vi "TEST.vi"() -> ()   [LabVIEW 2021]
uses:
  TEST ENNUM.ctl
  <vilib>/Instr/_visa.llb/VISA Configure Serial Port (Instr).vi
  <vilib>/Utility/file.llb/Write Delimited Spreadsheet (string).vi
  <vilib>/Utility/config.llb/NI_LVConfig.lvlib
  <vilib>/Utility/miscctls.llb/LVPointTypeDef.ctl
  Settings page.vi
  Exit Variable.vi
  Control 4.ctl
  <vilib>/Utility/config.llb/Write Key (Double).vi
panel:
  out "Printer":bool
  out "Part ID":string
  out "Printer Command":string
  out "TETS TYPE":string
  out "TETS MODE":string
  in  "Exit Button":bool
  in  "SETTINGS BUTTON 2":bool
  out "Communication Status":bool
  out "CH 1 FAIL":bool
  out "CH 10 FAIL":bool
  out "CH 10  PASS":bool
  out "CH 5 FAIL":bool
  out "CH 5 PASS":bool
  out "CH 4 FAIL":bool
  out "CH 4 PASS":bool
  out "CH 9 FAIL":bool
  out "CH 9 PASS":bool
  out "CH 8 FAIL":bool
  out "CH 8 PASS":bool
  out "CH 3 FAIL":bool
  out "CH 3 PASS":bool
  out "CH 2 FAIL":bool
  out "CH 2 PASS":bool
  out "CH 7 FAIL":bool
  out "CH 7 PASS":bool
  out "CH 6 FAIL":bool
  out "CH 6 PASS":bool
  out "CH 1 PASS":bool
  out "CH 10 RES VAL":string
  out "CH 10 STATUS":string
  out "CH 9 RES VAL":string
  out "CH 9 STATUS":string
  out "CH 8 RES VAL":string
  out "CH 8 STATUS":string
  out "CH 7 RES VAL":string
  out "CH 7 STATUS":string
  out "CH 6 RES VAL":string
  out "CH 6 STATUS":string
  out "CH 5 RES VAL":string
  out "CH 5 STATUS":string
  out "CH 4 RES VAL":string
  out "CH 4 STATUS":string
  out "CH 3 RES VAL":string
  out "CH 3 STATUS":string
  out "CH 2 RES VAL":string
  out "CH 2 STATUS":string
  out "Cancel Button":bool
  out "CH 1 RES VAL":string
  out "CH1 STATUS":string
  # "EOL TEST BENCH FOR THERMISTOR"
  # "Communication Status"
  # "Printer Communication Status"
  # "CHANNEL 5"
  # "CHANNEL 3"
  # "CHANNEL 4"
  # "CHANNEL 1"
  # "CHANNEL 2"
  # "STATUS"
  # "STATUS"
  # "STATUS"
  # "STATUS"
  # "STATUS"
  # "k Ohm"
  # "k Ohm"
  # "RESISTANCE VALUE"
  # "RESISTANCE VALUE"
  # "RESISTANCE VALUE"
  # "k Ohm"
  # "RESISTANCE VALUE"
  # "k Ohm"
  # "RESISTANCE VALUE"
  # "k Ohm"
  # "PASS"
  # "FAIL"
  # "PASS"
  # "FAIL"
  # "PASS"
  # "FAIL"
  # "PASS"
  # "FAIL"
  # "PASS"
  # "FAIL"
  # "QR DATA"
  # "CHANNEL 7"
  # "CHANNEL 6"
  # "CHANNEL 10"
  # "CHANNEL 8"
  # "CHANNEL 9"
  # "STATUS"
  # "STATUS"
  # "STATUS"
  # "STATUS"
  # "STATUS"
  # "RESISTANCE VALUE"
  # "RESISTANCE VALUE"
  # "k Ohm"
  # "RESISTANCE VALUE"
  # "k Ohm"
  # "RESISTANCE VALUE"
  # "k Ohm"
  # "k Ohm"
  # "RESISTANCE VALUE"
  # "k Ohm"
  # "PASS"
  # "FAIL"
  # "PASS"
  # "FAIL"
  # "PASS"
  # "FAIL"
  # "PASS"
  # "FAIL"
  # "PASS"
  # "FAIL"
  # "MODE :"
  # "TEST TYPE :"
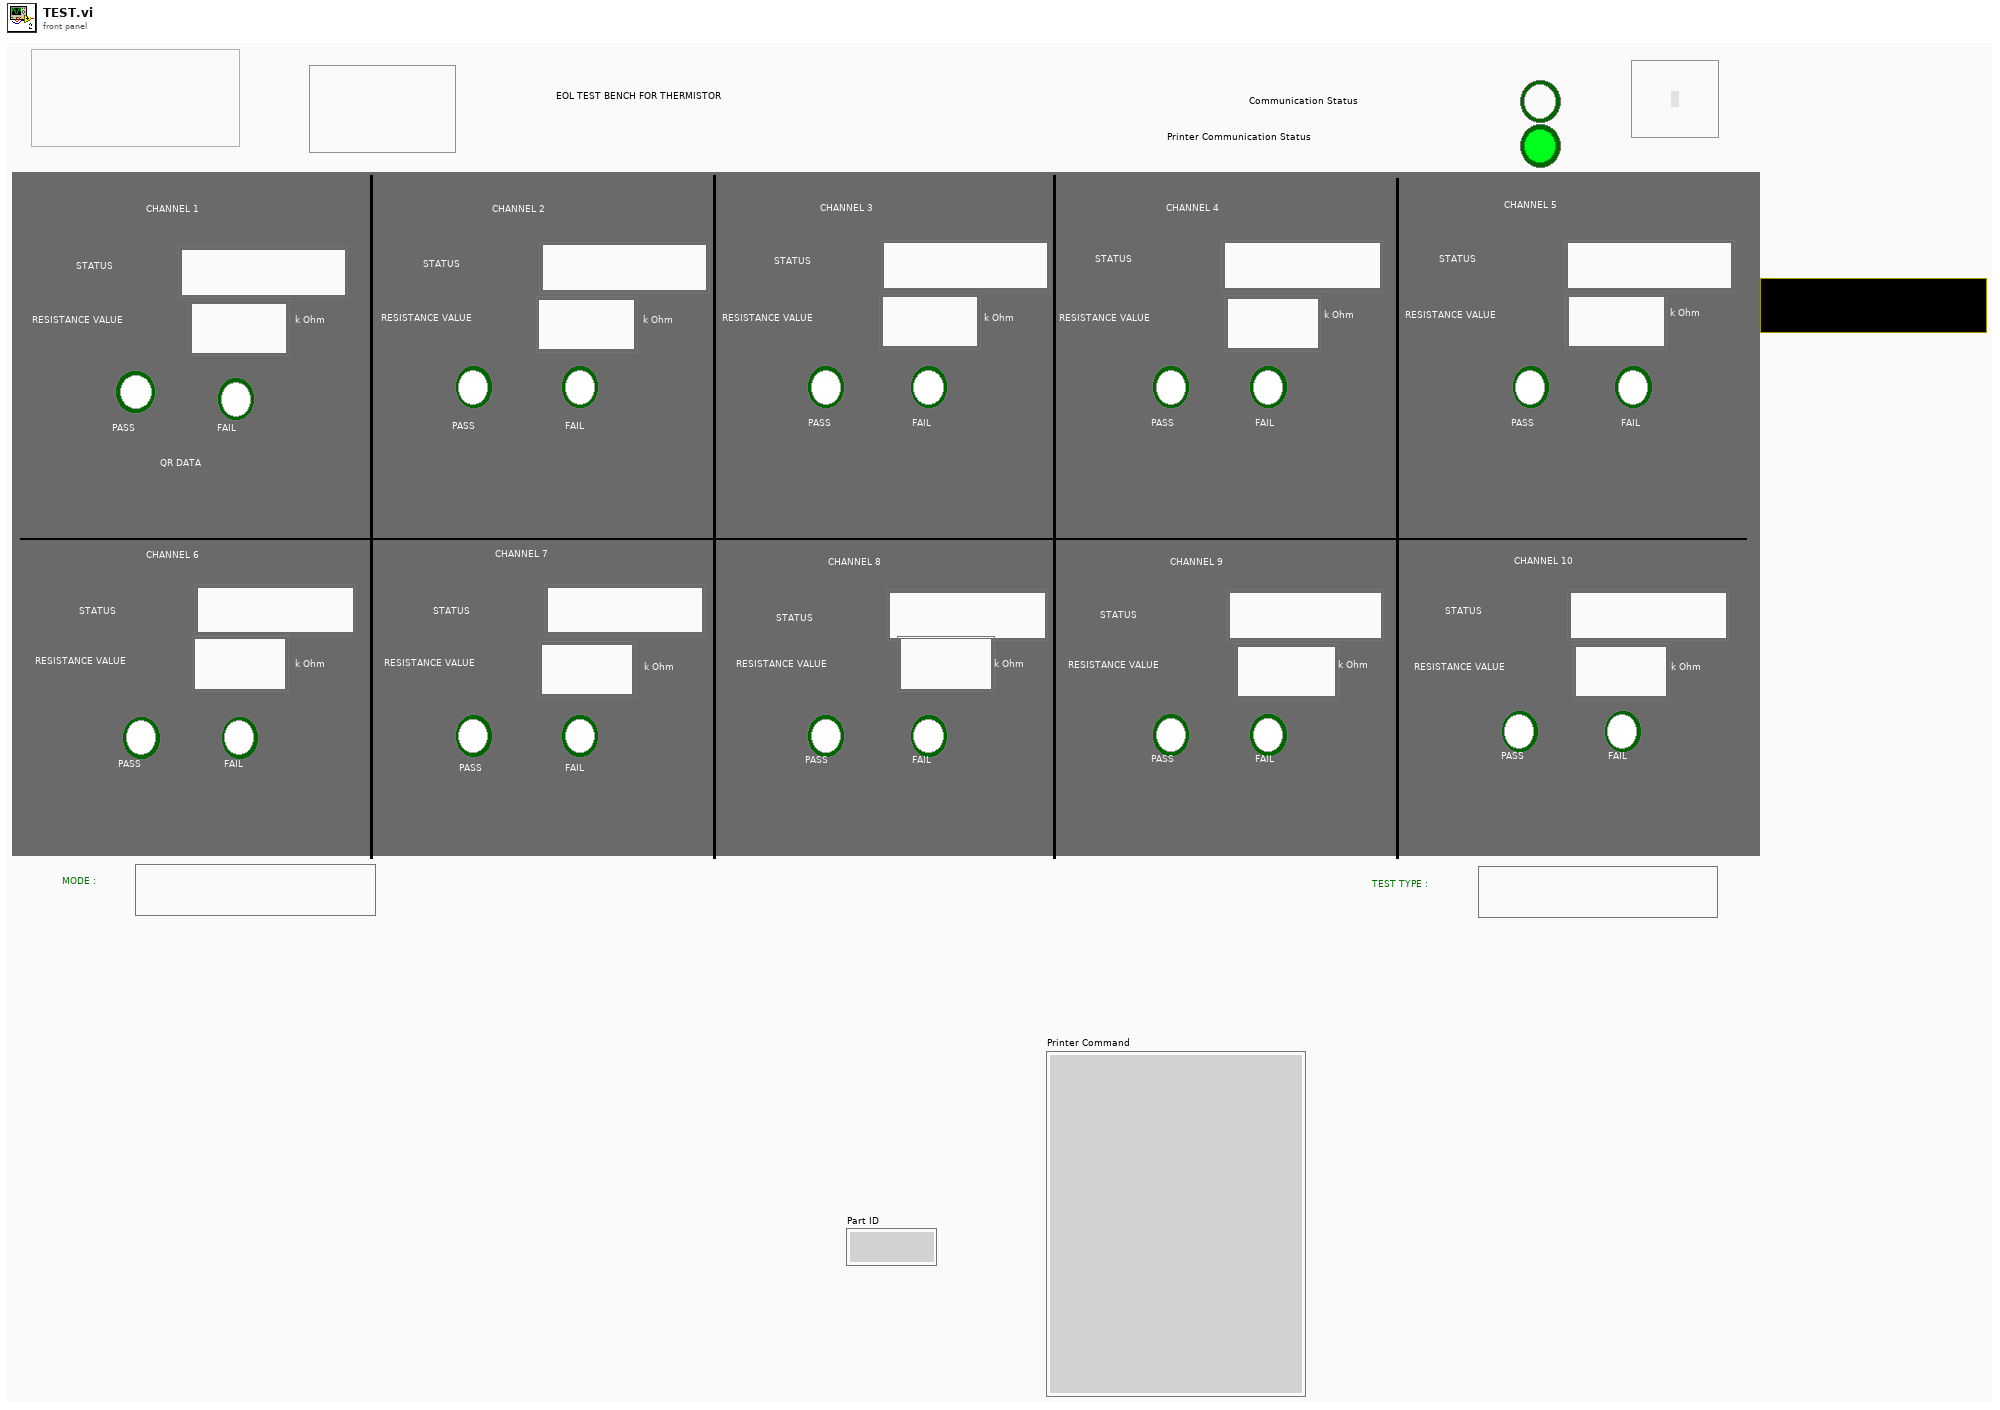
[diagram p1: front panel]
types:
  T1 = typedef "LVPointTypeDef.ctl" = cluster{"Horizontal":i16, "Vertical":i16}
  T2 = typedef "Control 4.ctl" = cluster{"VISA resource name":refnum<visa-resource-name>, "MODE":string, "PP 1":i32, "PP 2":i32, "PP 3":i32, "PP 4":i32, "PP 5":i32, "PP 6":i32, "PP 7":i32, "PP 8":i32, "PP 9":i32, "PP 10":i32, "CH  PASS  1":bool, "CH  PASS 2":bool, "CH  PASS 3":bool, "CH  PASS 4":bool, "CH  PASS 5":bool, "CH  PASS 6":bool, "CH  PASS 7":bool, "CH  PASS 8":bool, "CH  PASS 9":bool, "CH  PASS 10":bool, "CH  FAIL 1":bool, "CH  FAIL 2":bool, "CH  FAIL 3":bool, "CH  FAIL 4":bool, "CH  FAIL 5":bool, "CH  FAIL 6":bool, "CH  FAIL 7":bool, "CH  FAIL 8":bool, "CH  FAIL 9":bool, "CH  FAIL 10":bool, "RES VALUE 1":dbl, "RES VALUE 2":dbl, "RES VALUE 3":dbl, "RES VALUE 4":dbl, "RES VALUE 5":dbl, "RES VALUE 6":dbl, "RES VALUE 7":dbl, "RES VALUE 8":dbl, "RES VALUE 9":dbl, "RES VALUE 10":dbl, "SET VALUE 1":dbl, "SET VALUE 2":dbl, "SET VALUE 3":dbl, "SET VALUE 4":dbl, "SET VALUE 5":dbl, "SET VALUE 6":dbl, "SET VALUE 7":dbl, "SET VALUE 8":dbl, "SET VALUE 9":dbl, "SET VALUE 10":dbl, "TOL 1":dbl, "TOL 2":dbl, "TOL 3":dbl, "TOL 4":dbl, "TOL 5":dbl, "TOL 6":dbl, "TOL 7":dbl, "TOL 8":dbl, "TOL 9":dbl, "TOL 10":dbl, "START BIT":i32, "CH1 MIN TOL":dbl, "CH2 MIN TOL ":dbl, "CH3 MIN TOL ":dbl, "CH4 MIN TOL ":dbl, "CH5 MIN TOL ":dbl, "CH6 MIN TOL ":dbl, "CH7 MIN TOL  ":dbl, "CH8 MIN TOL  ":dbl, "CH9 MIN TOL   ":dbl, "CH10 MIN TOL   ":dbl, "CH1 MAX TOL ":dbl, "CH2 MAX TOL  ":dbl, "CH3 MAX TOL  ":dbl, "CH4 MAX TOL ":dbl, "CH5 MAX TOL  ":dbl, "CH6 MAX TOL  ":dbl, "CH7 MAX TOL   ":dbl, "CH8 MAX TOL  ":dbl, "CH9 MAX TOL    ":dbl, "CH10 MAX TOL   ":dbl}
  T3 = typedef "TEST ENNUM.ctl" = enum16{"TIMEOUT", "INITIALIZE", "CH SELECTION", "VALIDATING", "RESULT", "LED_SEQ", "READY TO PRINT", "REPORT ", "PART PRESENCE CHECKING"}
  T4 = typedef "NI_LVConfig.lvlib/Config Data RefNum.ctl" = refnum<k1>
  T5 = typedef "SERIAL N0.ctl" = string
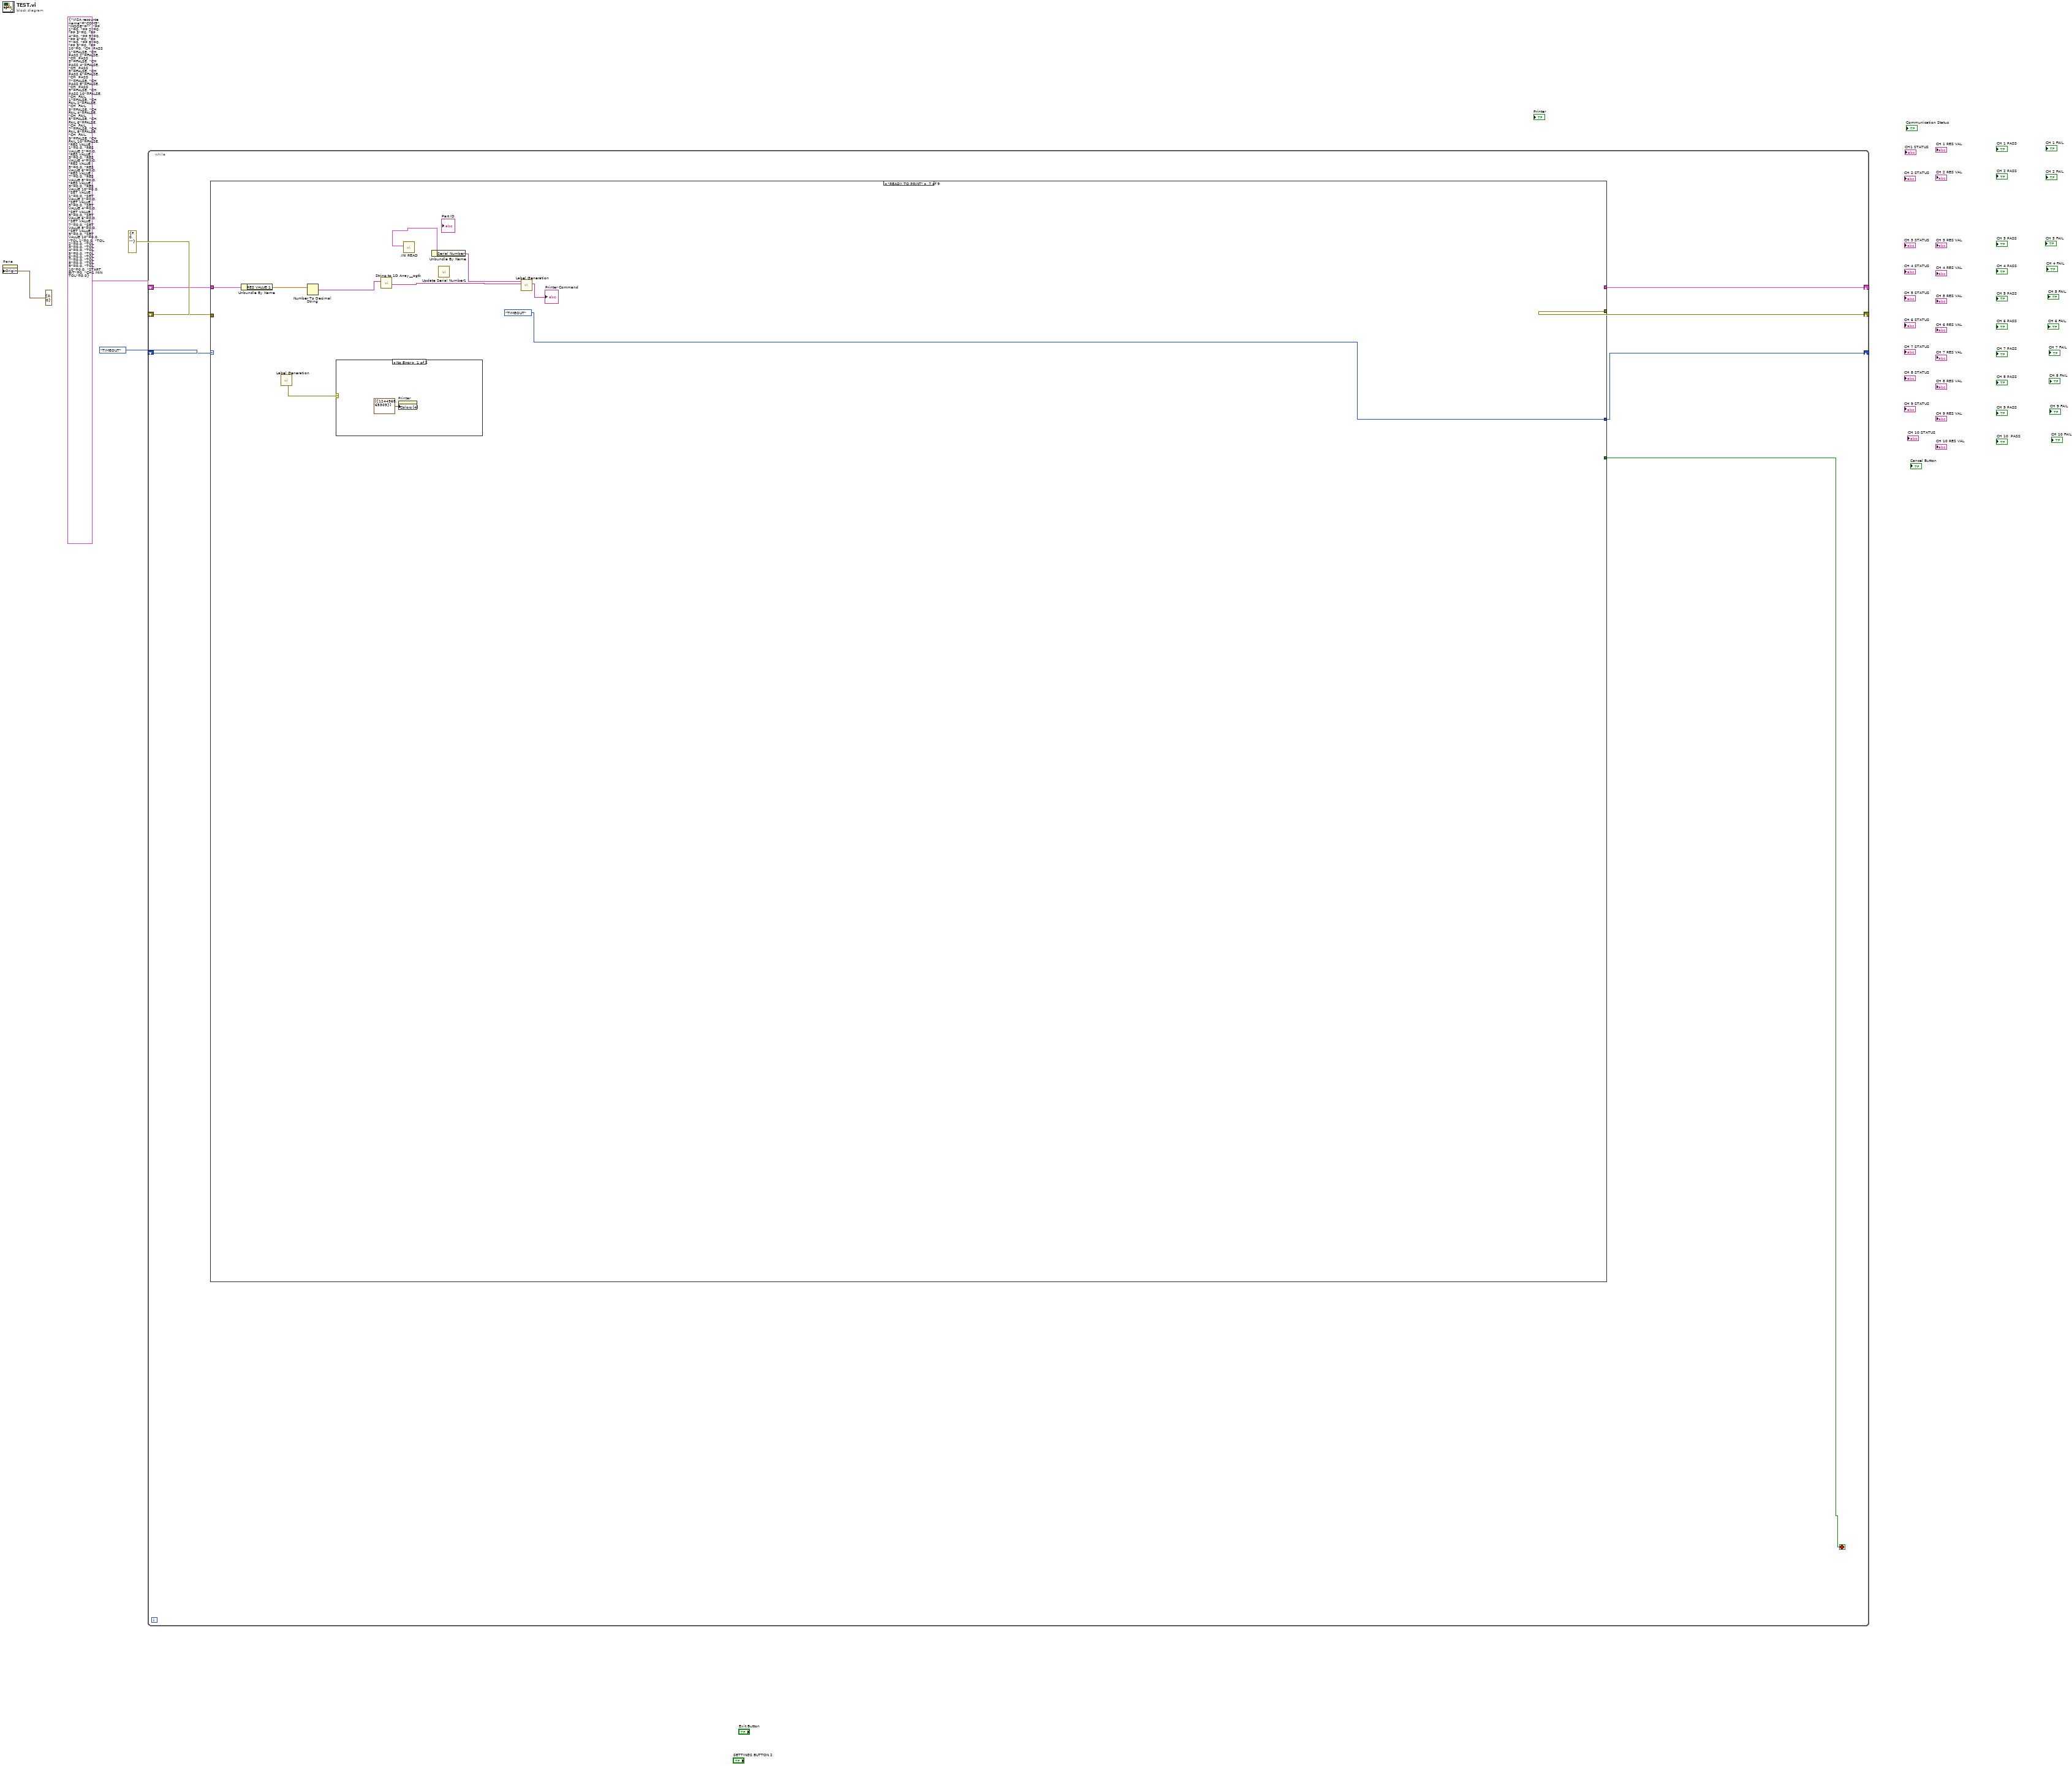
[diagram p0: block diagram]
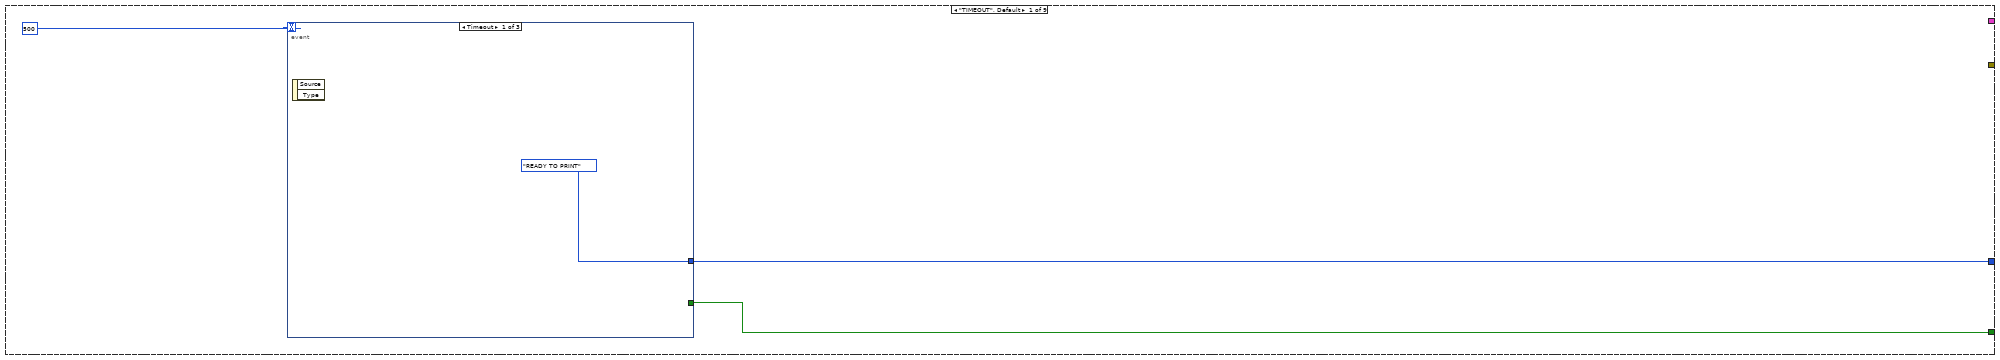
[diagram p2: hidden frame]
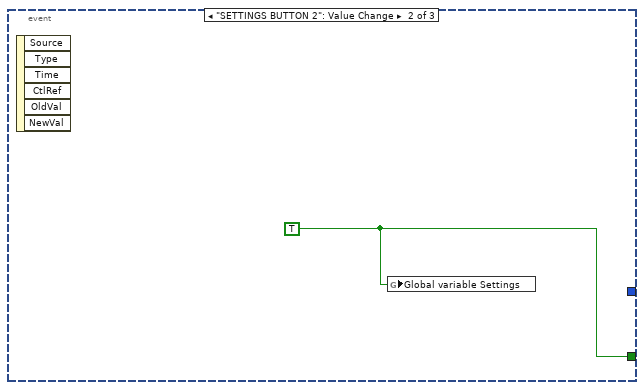
[diagram p3: hidden frame]
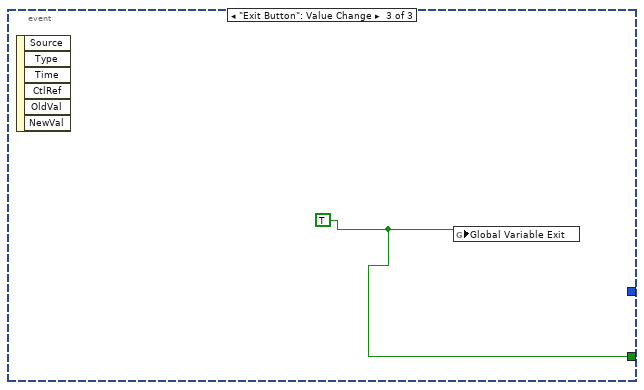
[diagram p4: hidden frame]
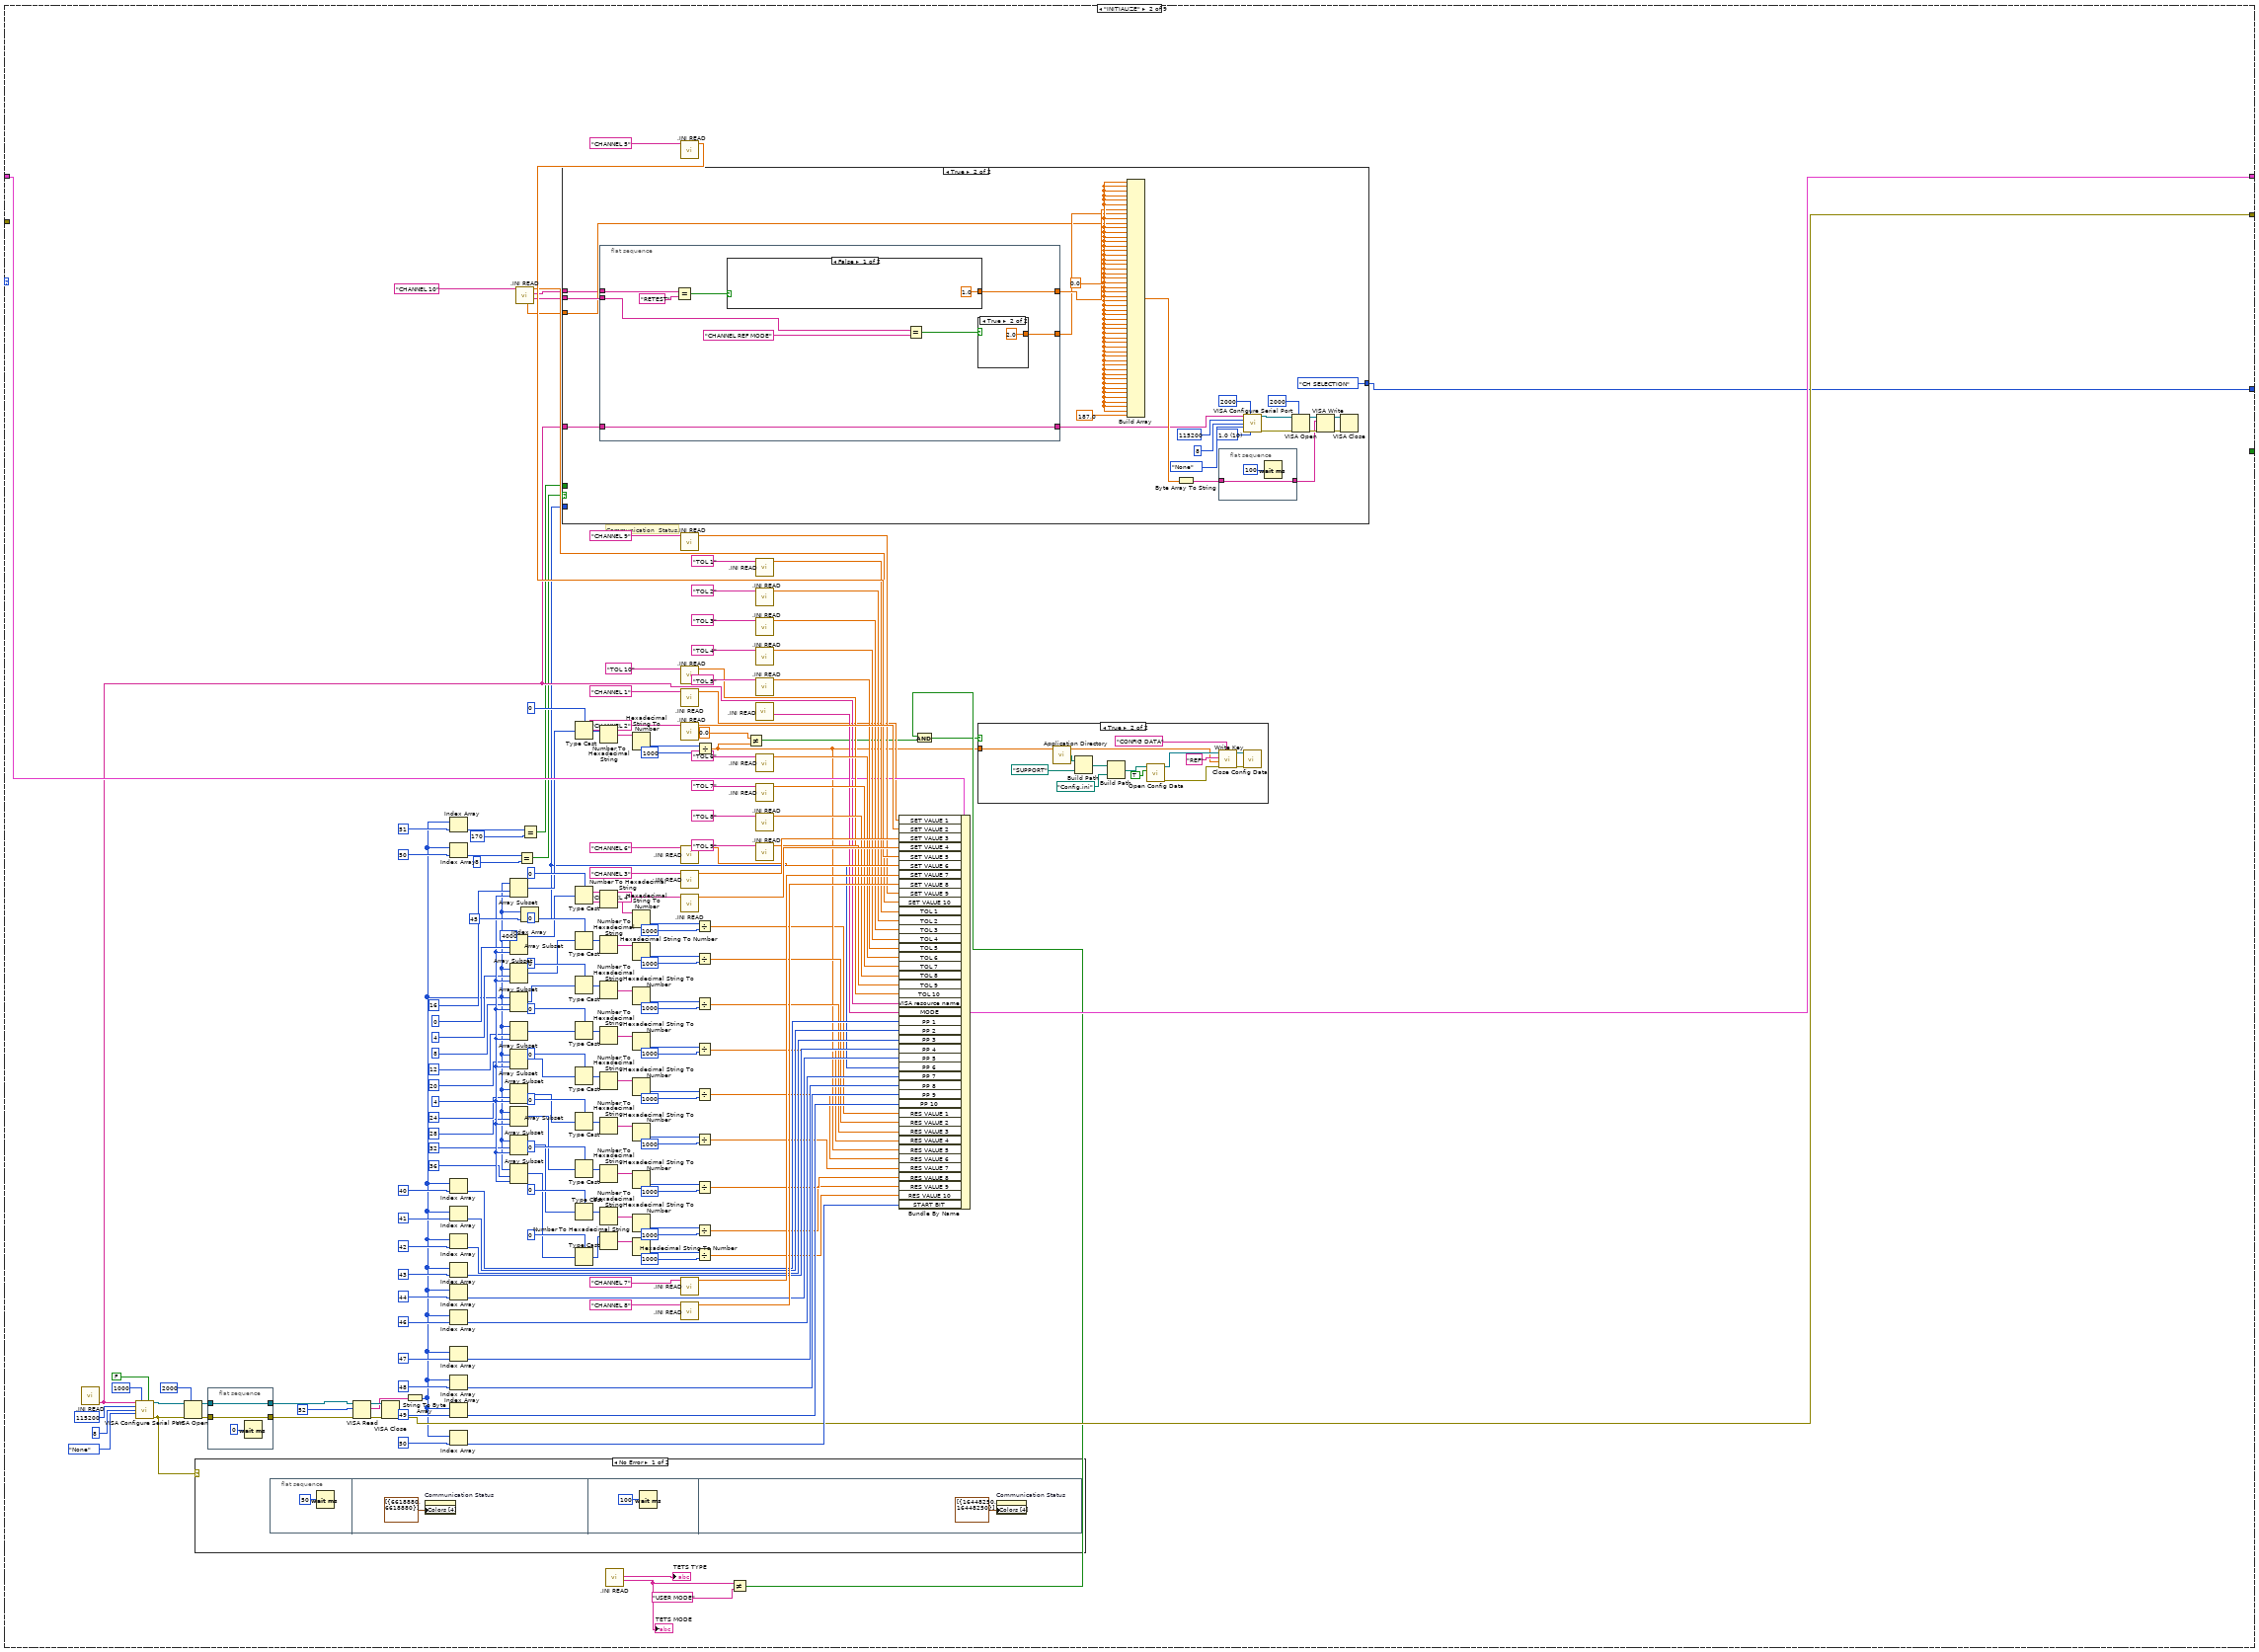
[diagram p5: hidden frame]
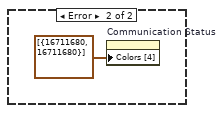
[diagram p7: hidden frame]
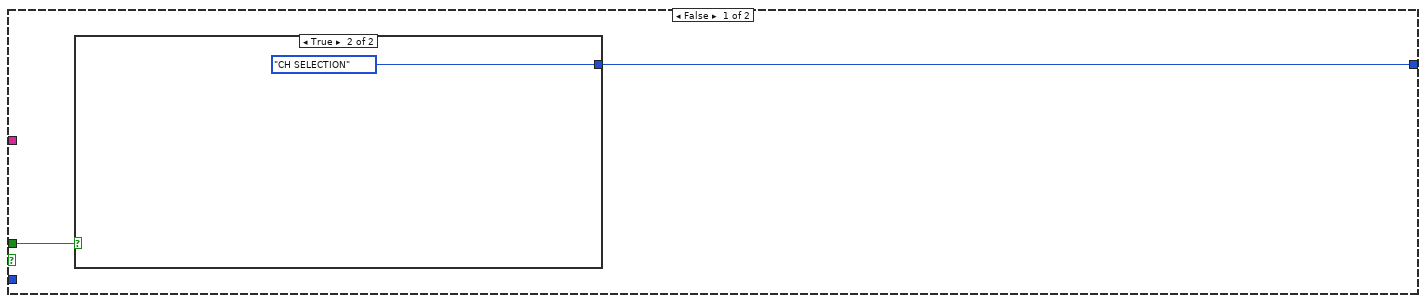
[diagram p8: hidden frame]
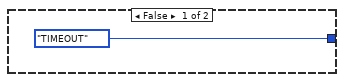
[diagram p9: hidden frame]
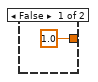
[diagram p10: hidden frame]
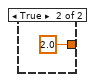
[diagram p11: hidden frame]
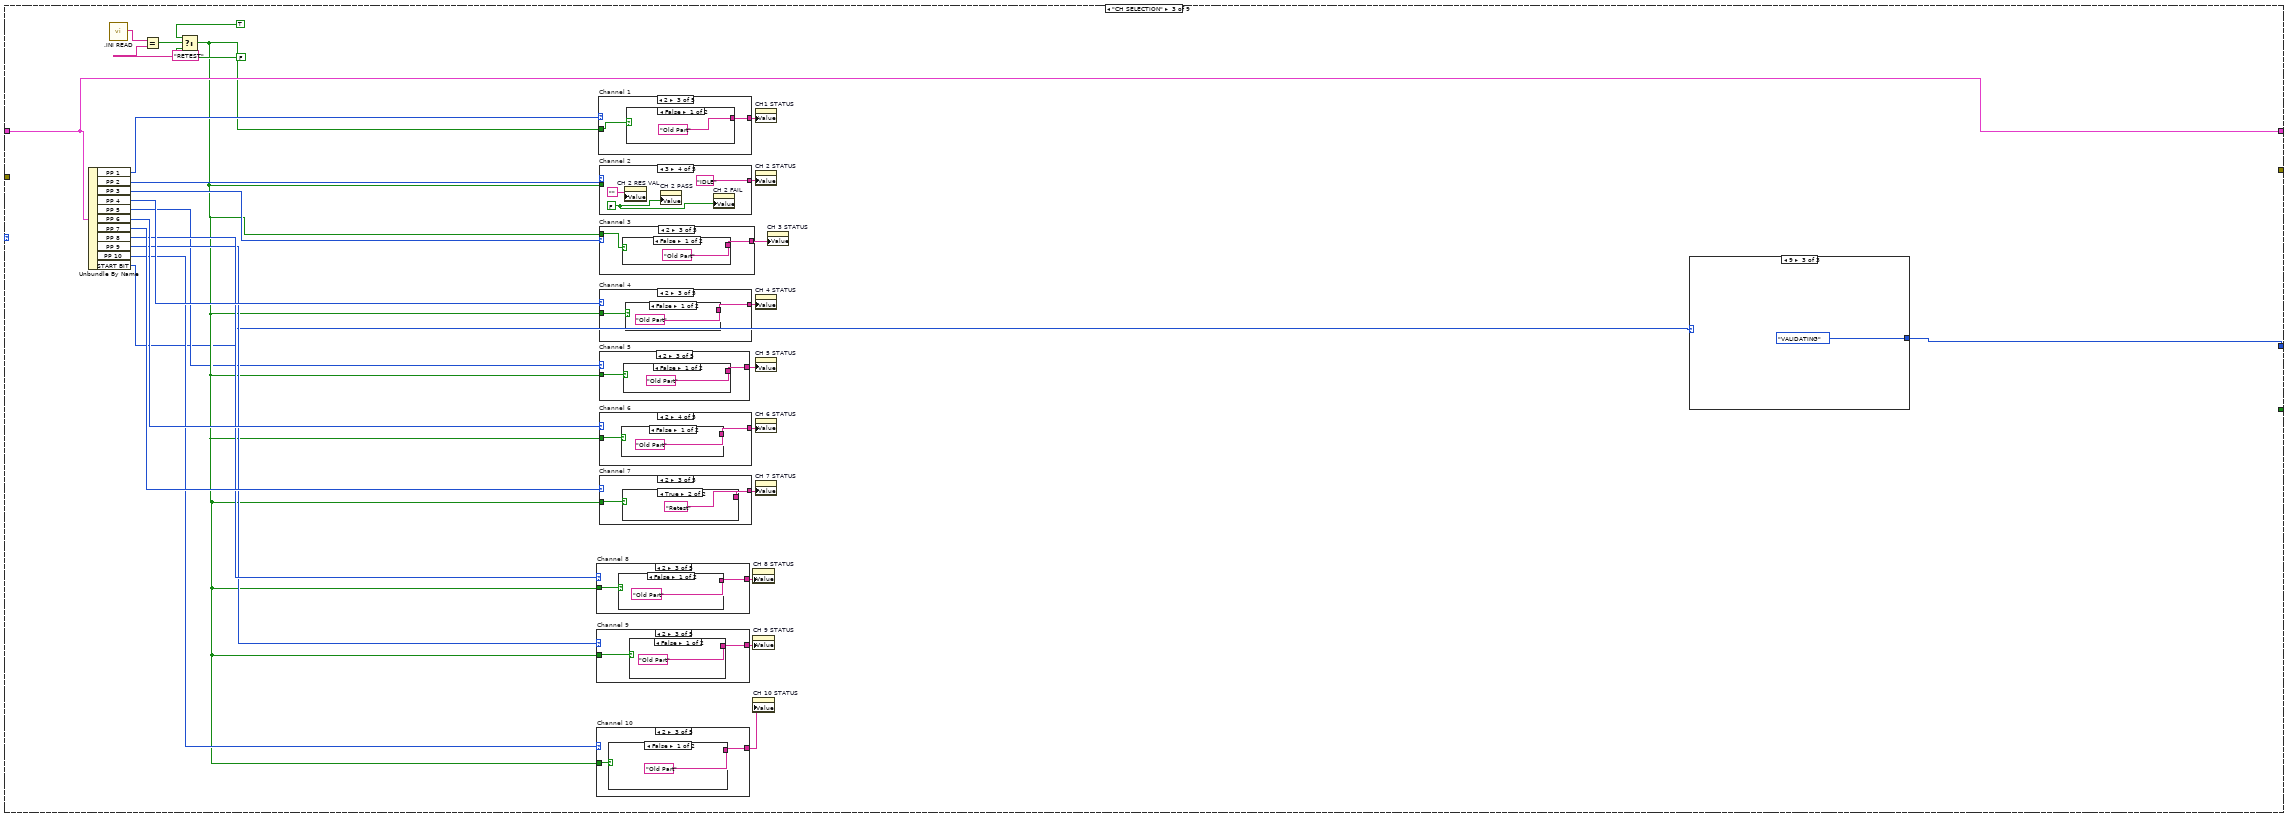
[diagram p12: hidden frame]
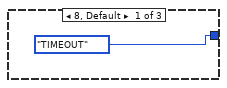
[diagram p13: hidden frame]
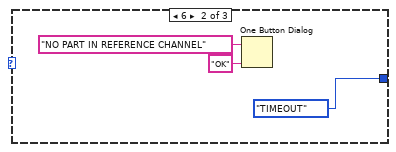
[diagram p14: hidden frame]
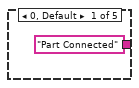
[diagram p15: hidden frame]
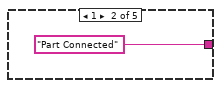
[diagram p16: hidden frame]
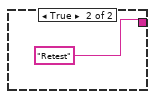
[diagram p17: hidden frame]
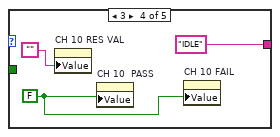
[diagram p18: hidden frame]
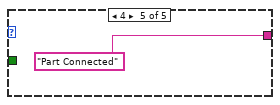
[diagram p19: hidden frame]
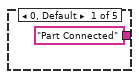
[diagram p20: hidden frame]
diagram:
  n1 = property on="Pane" class="Pane"("Origin"=T1 {"Horizontal"=0, "Vertical"=0}) -> ()  [unwired: 2 in, 2 out]
  n2 = while {
    shift-right: [w10] -> _
    shift-left: TEST_ENNUM."TIMEOUT" -> [w11]
    shift-right: [w9] -> _
    shift-left: T2 {"VISA resource name"="COM5", "MODE"="", "PP 1"=0, "PP 2"=0, "PP 3"=0, "PP 4"=0, "PP 5"=0, "PP 6"=0, "PP 7"=0, "PP 8"=0, "PP 9"=0, "PP 10"=0, "CH  PASS  1"=FALSE, "CH  PASS 2"=FALSE, "CH  PASS 3"=FALSE, "CH  PASS 4"=FALSE, "CH  PASS 5"=FALSE, "CH  PASS 6"=FALSE, "CH  PASS 7"=FALSE, "CH  PASS 8"=FALSE, "CH  PASS 9"=FALSE, "CH  PASS 10"=FALSE, "CH  FAIL 1"=FALSE, "CH  FAIL 2"=FALSE, "CH  FAIL 3"=FALSE, "CH  FAIL 4"=FALSE, "CH  FAIL 5"=FALSE, "CH  FAIL 6"=FALSE, "CH  FAIL 7"=FALSE, "CH  FAIL 8"=FALSE, "CH  FAIL 9"=FALSE, "CH  FAIL 10"=FALSE, "RES VALUE 1"=0.0, "RES VALUE 2"=0.0, "RES VALUE 3"=0.0, "RES VALUE 4"=0.0, "RES VALUE 5"=0.0, "RES VALUE 6"=0.0, "RES VALUE 7"=0.0, "RES VALUE 8"=0.0, "RES VALUE 9"=0.0, "RES VALUE 10"=0.0, "SET VALUE 1"=0.0, "SET VALUE 2"=0.0, "SET VALUE 3"=0.0, "SET VALUE 4"=0.0, "SET VALUE 5"=0.0, "SET VALUE 6"=0.0, "SET VALUE 7"=0.0, "SET VALUE 8"=0.0, "SET VALUE 9"=0.0, "SET VALUE 10"=0.0, "TOL 1"=0.0, "TOL 2"=0.0, "TOL 3"=0.0, "TOL 4"=0.0, "TOL 5"=0.0, "TOL 6"=0.0, "TOL 7"=0.0, "TOL 8"=0.0, "TOL 9"=0.0, "TOL 10"=0.0, "START BIT"=0, "CH1 MIN TOL"=0.0, "CH2 MIN TOL "=0.0, "CH3 MIN TOL "=0.0, "CH4 MIN TOL "=0.0, "CH5 MIN TOL "=0.0, "CH6 MIN TOL "=0.0, "CH7 MIN TOL  "=0.0, "CH8 MIN TOL  "=0.0, "CH9 MIN TOL   "=0.0, "CH10 MIN TOL   "=0.0, "CH1 MAX TOL "=0.0, "CH2 MAX TOL  "=0.0, "CH3 MAX TOL  "=0.0, "CH4 MAX TOL "=0.0, "CH5 MAX TOL  "=0.0, "CH6 MAX TOL  "=0.0, "CH7 MAX TOL   "=0.0, "CH8 MAX TOL  "=0.0, "CH9 MAX TOL    "=0.0, "CH10 MAX TOL   "=0.0} ("Cluster") -> [w7]
    shift-right: [w8] -> _
    shift-left: errorcluster {"status"=FALSE, "code"=0, "source"=""} ("error out") -> [w6]
    stop <- w5 stop-if-true
    n3 = case shown="\"READY TO PRINT\"" w11 {
      tunnel: [w13 w55 w267 TEST_ENNUM."RESULT" TEST_ENNUM."LED_SEQ" TEST_ENNUM."READY TO PRINT" TEST_ENNUM."TIMEOUT" TEST_ENNUM."TIMEOUT" _] -> w10
      tunnel: w7 -> [_ w141 w276 w423 w643 w862 w1024 w1035 _]
      tunnel: [_ w142 w276 w536 w643 w862 _ _ _] -> w9
      tunnel: [_ w59 _ _ _ w860 _ _ _] -> w8
      tunnel: w6 -> [_ _ _ _ _ _ _ _ _]
      tunnel: [w12 _ _ _ _ _ _ _ _] -> w5
      frame "TIMEOUT", Default {
        n4 = event shown="[0] Timeout" {
          selector: _ -> [_ _ _]
          dyn-events: _ -> [_ _ _]
          timeout: 500 -> [_ _ _]
          tunnel: [_ w16 w17] -> w12
          tunnel: [TEST_ENNUM."READY TO PRINT" _ _] -> w13
          event Timeout {
            n5 = event-data() -> ()  [unwired: 1 in, 2 out]
          }
          event "SETTINGS BUTTON 2": Value Change {
            w16 = TRUE
            n6 = event-data() -> ()  [unwired: 1 in, 6 out]
            n7 = global write "Settings page.vi" "Global variable Settings"(w16) -> ()
          }
          event "Exit Button": Value Change {
            w17 = TRUE
            n8 = event-data() -> ()  [unwired: 1 in, 6 out]
            n9 = global write "Exit Variable.vi" "Global Variable Exit"(w17) -> ()
          }
        }
      }
      frame "INITIALIZE" {
        w139 = 4 ("length")
        # "Communication  Status"
        n10 = call ".INI READ.vi"() -> ("COM"=w56:string)  [unwired: 4 in, 7 out]
        n11 = call-poly "VISA Configure Serial Port"("VISA resource name"=w56, "timeout (10sec)"=u32 1000, "Enable Termination\nChar (T)"=FALSE ("Enable Termination\nChar (T)"), "baud rate (9600)"=u32 115200, "data bits (8)"=u16 8, "parity (0:none)"=enum16{"None", "Odd", "Even", "Mark", "Space"}."None") -> ("VISA resource name out"=w46:refnum<visa-resource-name>, "error out"=w61:errorcluster)  [unwired: 8 in]
        n12 = VISA Open(timeout (0)=u32 2000 ("VISA Open timeout (0)"), error in (no error)=w61, VISA resource name=w46) -> (VISA resource name=w38:refnum<visa-resource-name>, error out=w40:errorcluster)  [unwired: 2 in]
        n13 = case shown="No Error" w61 {
          frame No Error {
            n14 = flat-sequence {
              frame #0 {
                n15 = Wait (ms)(milliseconds to wait=u32 50) -> ()  [unwired: 1 out]
              }
              frame #1 {
                n16 = property on="Communication Status" class="Bool (strict)"("Colors [4]"=cluster{u32, u32}[] [{6618880, 6618880}]) -> ()  [unwired: 2 in, 2 out]
              }
              frame #2 {
                n17 = Wait (ms)(milliseconds to wait=u32 100) -> ()  [unwired: 1 out]
              }
              frame #3 {
                n18 = property on="Communication Status" class="Bool (strict)"("Colors [4]"=cluster{u32, u32}[] [{16448250, 16448250}]) -> ()  [unwired: 2 in, 2 out]
              }
            }
          }
          frame Error {
            n19 = property on="Communication Status" class="Bool (strict)"("Colors [4]"=cluster{u32, u32}[] [{16711680, 16711680}]) -> ()  [unwired: 2 in, 2 out]
          }
        }
        n20 = flat-sequence {
          tunnel: [w217] -> w41
          tunnel: w40 -> [w217]
          tunnel: [w216] -> w39
          tunnel: w38 -> [w216]
          frame #0 {
            n21 = Wait (ms)(milliseconds to wait=u32 0) -> ()  [unwired: 1 out]
          }
        }
        n22 = VISA Read(VISA resource name=w39, byte count=u32 52, error in (no error)=w41) -> (VISA resource name out=w42:refnum<visa-resource-name>, read buffer=w36:string, error out=w37:errorcluster)  [unwired: 1 out]
        n23 = VISA Close(VISA resource name=w42, error in (no error)=w37) -> (error out=w59:errorcluster)
        n24 = String To Byte Array(string=w36) -> (unsigned byte array=w28:u8[])
        n25 = Index Array(array=w28, index=51) -> (element=w57:u8)
        n26 = Index Array(array=w28, index=50) -> (element=w52:u8)
        n27 = Index Array(array=w28, index=40) -> (element=w151:u8)
        n28 = Index Array(array=w28, index=41) -> (element=w150:u8)
        n29 = Index Array(array=w28, index=42) -> (element=w149:u8)
        n30 = Index Array(array=w28, index=43) -> (element=w148:u8)
        n31 = Index Array(array=w28, index=44) -> (element=w147:u8)
        n32 = Index Array(array=w28, index=46) -> (element=w146:u8)
        n33 = Index Array(array=w28, index=47) -> (element=w145:u8)
        n34 = Index Array(array=w28, index=48) -> (element=w144:u8)
        n35 = Index Array(array=w28, index=49) -> (element=w143:u8)
        n36 = Index Array(array=w28, index=50) -> (element=w60:u8)
        n37 = Array Subset(array=w28, index=16, length=w139) -> (w109:u8[])
        n38 = Array Subset(array=w28, index=0, length=w139) -> ()  [unwired: 1 out]
        n39 = Array Subset(array=w28, index=4, length=w139) -> (w117:u8[])
        n40 = Array Subset(array=w28, index=8, length=w139) -> (w18:u8[])
        n41 = Array Subset(array=w28, index=12, length=w139) -> (w112:u8[])
        n42 = Array Subset(array=w28, index=20, length=w139) -> (w106:u8[])
        n43 = Array Subset(array=w28, index=24, length=w139) -> (w103:u8[])
        n44 = Array Subset(array=w28, index=28, length=w139) -> (w100:u8[])
        n45 = Array Subset(array=w28, index=32, length=w139) -> (w97:u8[])
        n46 = Array Subset(array=w28, index=36, length=w139) -> (w94:u8[])
        n47 = call ".INI READ.vi"("KEY"="CHANNEL 10") -> ("MODE"=w24:string, "TEST MODE"=w23:string, "OUT"=w183:dbl, "TIME"=w25:dbl)  [unwired: 3 in, 4 out]
        n48 = Equal?(x=w52, y=u8 8) -> (x = y?=w50:bool)
        n49 = Index Array(array=w28, index=45) -> (element=w26:u8)
        n50 = Equal?(x=w57, y=u8 170) -> (x = y?=w53:bool)
        n51 = case shown="True" w50 {
          tunnel: w56 -> [_ w231]
          tunnel: [w223 TEST_ENNUM."CH SELECTION"] -> w55
          tunnel: w53 -> [w224 _]
          tunnel: w26 -> [_ _]
          tunnel: w24 -> [_ w229]
          tunnel: w25 -> [_ w228]
          tunnel: w23 -> [_ w227]
          frame False {
            n52 = case shown="True" w224 {
              tunnel: [TEST_ENNUM."TIMEOUT" TEST_ENNUM."CH SELECTION"] -> w223
              frame False {
              }
              frame True {
              }
            }
          }
          frame True {
            w244 = u16 10 items=["1.0"=10, "1.5"=15, "2.0"=20] ("stop bits (10: 1 bit)")
            w235 = 0.0 ("element")
            n53 = flat-sequence {
              tunnel: [w258] -> w233
              tunnel: [w255] -> w232
              tunnel: w231 -> [w254]
              tunnel: [w254] -> w230
              tunnel: w229 -> [w253]
              tunnel: w227 -> [w252]
              frame #0 {
                n54 = Equal?(x=w252, y="RETEST") -> (x = y?=w259:bool)
                n55 = case shown="False" w259 {
                  tunnel: [1.0 ("element") 2.0 ("element")] -> w258
                  frame False {
                  }
                  frame True {
                  }
                }
                n56 = Equal?(x=w253, y="CHANNEL REF MODE") -> (x = y?=w256:bool)
                n57 = case shown="True" w256 {
                  tunnel: [1.0 ("element") 2.0 ("element")] -> w255
                  frame False {
                  }
                  frame True {
                  }
                }
              }
            }
            n58 = Build Array(w235, w235, w235, w235, w235, w235, w233, w232, w235, w228, w235, w235, w235, w235, w235, w235, w235, w235, w235, w235, w235, w235, w235, w235, w235, w235, w235, w235, w235, w235, w235, w235, w235, w235, w235, w235, w235, w235, w235, w235, w235, w235, w235, w235, w235, w235, w235, w235, w235, w235, w235, 187.0 ("element")) -> (w251:dbl[])
            n59 = Byte Array To String(unsigned byte array=w251) -> (string=w237:string)
            n60 = flat-sequence {
              tunnel: w237 -> [w266]
              tunnel: [w266] -> w236
              frame #0 {
                n61 = Wait (ms)(milliseconds to wait=u32 100) -> ()  [unwired: 1 out]
              }
            }
            n62 = call-poly "VISA Configure Serial Port"("VISA resource name"=w230, "timeout (10sec)"=u32 2000, "baud rate (9600)"=u32 115200, "data bits (8)"=u16 8, "parity (0:none)"=enum16{"None", "Odd", "Even", "Mark", "Space"}."None", "stop bits (10: 1 bit)"=w244) -> ("VISA resource name out"=w250:refnum<visa-resource-name>, "error out"=w249:errorcluster)  [unwired: 8 in]
            n63 = VISA Open(timeout (0)=u32 2000 ("VISA Open timeout (0)"), error in (no error)=w249, VISA resource name=w250) -> (VISA resource name=w243:refnum<visa-resource-name>, error out=w242:errorcluster)  [unwired: 2 in]
            n64 = VISA Write(VISA resource name=w243, write buffer=w236, error in (no error)=w242) -> (VISA resource name out=w240:refnum<visa-resource-name>, error out=w239:errorcluster)  [unwired: 1 out]
            n65 = VISA Close(VISA resource name=w240, error in (no error)=w239) -> ()  [unwired: 1 out]
          }
        }
        n66 = Type Cast(type=0 ("index"), x=w109) -> (*(type *) &x=w108:i32)
        n67 = Type Cast(type=0 ("index"), x=4000) -> (*(type *) &x=w119:i32)
        n68 = Type Cast(type=0 ("index"), x=w117) -> (*(type *) &x=w116:i32)
        n69 = Type Cast(type=0 ("index"), x=w18) -> (*(type *) &x=w114:i32)
        n70 = Type Cast(type=0 ("index"), x=w112) -> (*(type *) &x=w111:i32)
        n71 = Type Cast(type=0 ("index"), x=w106) -> (*(type *) &x=w105:i32)
        n72 = Type Cast(type=0 ("index"), x=w103) -> (*(type *) &x=w102:i32)
        n73 = Type Cast(type=0 ("index"), x=w100) -> (*(type *) &x=w99:i32)
        n74 = Type Cast(type=0 ("index"), x=w97) -> (*(type *) &x=w96:i32)
        n75 = Type Cast(type=0 ("index"), x=w94) -> (*(type *) &x=w93:i32)
        n76 = Number To Hexadecimal String(2:w108) -> (0:w107:string)  [unwired: 1 in]
        n77 = Number To Hexadecimal String(2:w119) -> (0:w118:string)  [unwired: 1 in]
        n78 = Number To Hexadecimal String(2:w116) -> (0:w115:string)  [unwired: 1 in]
        n79 = Number To Hexadecimal String(2:w114) -> (0:w113:string)  [unwired: 1 in]
        n80 = Number To Hexadecimal String(2:w111) -> (0:w110:string)  [unwired: 1 in]
        n81 = Number To Hexadecimal String(2:w105) -> (0:w104:string)  [unwired: 1 in]
        n82 = Number To Hexadecimal String(2:w102) -> (0:w101:string)  [unwired: 1 in]
        n83 = Number To Hexadecimal String(2:w99) -> (0:w98:string)  [unwired: 1 in]
        n84 = Number To Hexadecimal String(2:w96) -> (0:w95:string)  [unwired: 1 in]
        n85 = Number To Hexadecimal String(2:w93) -> (0:w92:string)  [unwired: 1 in]
        n86 = call ".INI READ.vi"() -> ("MODE"=w22:string, "TEST MODE"=→"TETS TYPE":string)  [unwired: 4 in, 6 out]
        "TETS MODE" <- w22
        n87 = Hexadecimal String To Number(string=w107) -> (number=w80:u32)  [unwired: 2 in, 1 out]
        n88 = Hexadecimal String To Number(string=w118) -> (number=w91:u32)  [unwired: 2 in, 1 out]
        n89 = Hexadecimal String To Number(string=w115) -> (number=w88:u32)  [unwired: 2 in, 1 out]
        n90 = Hexadecimal String To Number(string=w113) -> (number=w86:u32)  [unwired: 2 in, 1 out]
        n91 = Hexadecimal String To Number(string=w110) -> (number=w83:u32)  [unwired: 2 in, 1 out]
        n92 = Hexadecimal String To Number(string=w104) -> (number=w65:u32)  [unwired: 2 in, 1 out]
        n93 = Hexadecimal String To Number(string=w101) -> (number=w77:u32)  [unwired: 2 in, 1 out]
        n94 = Hexadecimal String To Number(string=w98) -> (number=w74:u32)  [unwired: 2 in, 1 out]
        n95 = Hexadecimal String To Number(string=w95) -> (number=w71:u32)  [unwired: 2 in, 1 out]
        n96 = Hexadecimal String To Number(string=w92) -> (number=w68:u32)  [unwired: 2 in, 1 out]
        n97 = call ".INI READ.vi"("KEY"="CHANNEL 5") -> ("OUT"=w188:dbl)  [unwired: 3 in, 7 out]
        n98 = call ".INI READ.vi"("KEY"="CHANNEL 9") -> ("OUT"=w184:dbl)  [unwired: 3 in, 7 out]
        n99 = call ".INI READ.vi"("KEY"="TOL 10") -> ("OUT"=w163:dbl)  [unwired: 3 in, 7 out]
        n100 = call ".INI READ.vi"("KEY"="CHANNEL 1") -> ("OUT"=w33:dbl)  [unwired: 3 in, 7 out]
        n101 = call ".INI READ.vi"("KEY"="CHANNEL 2") -> ("OUT"=w191:dbl)  [unwired: 3 in, 7 out]
        n102 = call ".INI READ.vi"("KEY"="CHANNEL 6") -> ("OUT"=w187:dbl)  [unwired: 3 in, 7 out]
        n103 = call ".INI READ.vi"("KEY"="CHANNEL 3") -> ("OUT"=w190:dbl)  [unwired: 3 in, 7 out]
        n104 = call ".INI READ.vi"("KEY"="CHANNEL 4") -> ("OUT"=w189:dbl)  [unwired: 3 in, 7 out]
        n105 = call ".INI READ.vi"("KEY"="CHANNEL 7") -> ("OUT"=w186:dbl)  [unwired: 3 in, 7 out]
        n106 = call ".INI READ.vi"("KEY"="CHANNEL 8") -> ("OUT"=w185:dbl)  [unwired: 3 in, 7 out]
        n107 = Divide(x=w91, y=u32 1000) -> (x/y=w20:dbl)
        n108 = Divide(x=w88, y=u32 1000) -> (x/y=w87:dbl)
        n109 = Divide(x=w86, y=u32 1000) -> (x/y=w84:dbl)
        n110 = Divide(x=w83, y=u32 1000) -> (x/y=w81:dbl)
        n111 = Divide(x=w65, y=u32 1000) -> (x/y=w78:dbl)
        n112 = Divide(x=w77, y=u32 1000) -> (x/y=w75:dbl)
        n113 = Divide(x=w74, y=u32 1000) -> (x/y=w72:dbl)
        n114 = Divide(x=w71, y=u32 1000) -> (x/y=w69:dbl)
        n115 = Divide(x=w68, y=u32 1000) -> (x/y=w63:dbl)
        n116 = Divide(x=w80, y=u32 1000) -> (x/y=w27:dbl)
        n117 = Not Equal?(x=w22, y="USER MODE") -> (x != y?=w30:bool)
        n118 = Not Equal?(x=0.0, y=w27) -> (x != y?=w31:bool)
        n119 = call ".INI READ.vi"() -> ("MODE"=w162:string)  [unwired: 4 in, 7 out]
        n120 = call ".INI READ.vi"("KEY"="TOL 1") -> ("OUT"=w172:dbl)  [unwired: 3 in, 7 out]
        n121 = call ".INI READ.vi"("KEY"="TOL 2") -> ("OUT"=w171:dbl)  [unwired: 3 in, 7 out]
        n122 = call ".INI READ.vi"("KEY"="TOL 3") -> ("OUT"=w170:dbl)  [unwired: 3 in, 7 out]
        n123 = call ".INI READ.vi"("KEY"="TOL 4") -> ("OUT"=w169:dbl)  [unwired: 3 in, 7 out]
        n124 = call ".INI READ.vi"("KEY"="TOL 5") -> ("OUT"=w168:dbl)  [unwired: 3 in, 7 out]
        n125 = call ".INI READ.vi"("KEY"="TOL 6") -> ("OUT"=w167:dbl)  [unwired: 3 in, 7 out]
        n126 = call ".INI READ.vi"("KEY"="TOL 7") -> ("OUT"=w166:dbl)  [unwired: 3 in, 7 out]
        n127 = call ".INI READ.vi"("KEY"="TOL 8") -> ("OUT"=w165:dbl)  [unwired: 3 in, 7 out]
        n128 = call ".INI READ.vi"("KEY"="TOL 9") -> ("OUT"=w164:dbl)  [unwired: 3 in, 7 out]
        n129 = Bundle By Name(cluster=w141, "SET VALUE 1"=w33, "SET VALUE 2"=w191, "SET VALUE 3"=w190, "SET VALUE 4"=w189, "SET VALUE 5"=w188, "SET VALUE 6"=w187, "SET VALUE 7"=w186, "SET VALUE 8"=w185, "SET VALUE 9"=w184, "SET VALUE 10"=w183, "TOL 1"=w172, "TOL 2"=w171, "TOL 3"=w170, "TOL 4"=w169, "TOL 5"=w168, "TOL 6"=w167, "TOL 7"=w166, "TOL 8"=w165, "TOL 9"=w164, "TOL 10"=w163, "VISA resource name"=w56, "MODE"=w162, "PP 1"=w151, "PP 2"=w150, "PP 3"=w149, "PP 4"=w148, "PP 5"=w147, "PP 6"=w26, "PP 7"=w146, "PP 8"=w145, "PP 9"=w144, "PP 10"=w143, "RES VALUE 1"=w20, "RES VALUE 2"=w87, "RES VALUE 3"=w84, "RES VALUE 4"=w81, "RES VALUE 5"=w27, "RES VALUE 6"=w78, "RES VALUE 7"=w75, "RES VALUE 8"=w72, "RES VALUE 9"=w69, "RES VALUE 10"=w63, "START BIT"=w60) -> (w142:T2)
        n130 = And(x=w30, y=w31) -> (x .and. y?=w29:bool)
        n131 = case shown="True" w29 {
          tunnel: w27 -> [_ w202]
          frame False {
          }
          frame True {
            n132 = call <vilib>:"Application Directory.vi"() -> ("Application Directory"=w213:path)
            n133 = Build Path(base path=w213, name or relative path=path "SUPPORT") -> (appended path=w214:path)
            n134 = Build Path(base path=w214, name or relative path=path "Config.ini") -> (appended path=w210:path)
            n135 = call <vilib>:"Open Config Data.vi"("create file if necessary (T)"=TRUE, "configuration file path"=w210) -> ("error out"=w203:errorcluster, "refnum"=w208:T4)  [unwired: 7 in, 1 out]
            n136 = call-poly <vilib>:"Write Key.vi"("section"="CONFIG DATA", "error in (no error)"=w203, "value"=w202, "key"="REF", "refnum"=w208) -> ("error out"=w204:errorcluster, "refnum out"=w205:T4)  [unwired: 4 in, 1 out]
            n137 = call <vilib>:"Close Config Data.vi"("error in (no error)"=w204, "refnum"=w205) -> ()  [unwired: 8 in, 2 out]
          }
        }
      }
      frame "CH SELECTION" {
        n138 = Unbundle By Name(w276) -> ("PP 1"=w295:i32, "PP 2"=w284:i32, "PP 3"=w283:i32, "PP 4"=w282:i32, "PP 5"=w269:i32, "PP 6"=w281:i32, "PP 7"=w280:i32, "PP 8"=w279:i32, "PP 9"=w278:i32, "PP 10"=w277:i32, "START BIT"=w268:i32)
        n139 = call ".INI READ.vi"() -> ("TEST MODE"=w275:string)  [unwired: 4 in, 7 out]
        n140 = Equal?(x=w275, y="RETEST") -> (x = y?=w273:bool)
        n141 = Select(t=TRUE, s=w273, f=FALSE) -> (s? t:f=w270:bool)
        n142 = case "Channel 8" shown="2" w279 {
          tunnel: ["Part Connected" "Part Connected" w324 "IDLE" "Part Conected"] -> w287
          tunnel: w270 -> [_ _ w323 _ _]
          frame 0, Default {
          }
          frame 1 {
          }
          frame 2 {
            n143 = case shown="False" w323 {
              tunnel: ["Old Part" "Retest"] -> w324
              frame False {
              }
              frame True {
              }
            }
          }
          frame 3 {
            w328 = FALSE
            n144 = property on="CH 8 RES VAL" class="Str"("Value"="") -> ()  [unwired: 2 in, 2 out]
            n145 = property on="CH 8 PASS" class="Bool (strict)"("Value"=w328) -> ()  [unwired: 2 in, 2 out]
            n146 = property on="CH 8 FAIL" class="Bool (strict)"("Value"=w328) -> ()  [unwired: 2 in, 2 out]
          }
          frame 4 {
          }
        }
        n147 = case "Channel 9" shown="2" w278 {
          tunnel: ["Part Connected" "Part Connected" w314 "IDLE" "Part Connected"] -> w286
          tunnel: w270 -> [_ _ w313 _ _]
          frame 0, Default {
          }
          frame 1 {
          }
          frame 2 {
            n148 = case shown="False" w313 {
              tunnel: ["Old Part" "Retest"] -> w314
              frame False {
              }
              frame True {
              }
            }
          }
          frame 3 {
            w318 = FALSE
            n149 = property on="CH 9 RES VAL" class="Str"("Value"="") -> ()  [unwired: 2 in, 2 out]
            n150 = property on="CH 9 PASS" class="Bool (strict)"("Value"=w318) -> ()  [unwired: 2 in, 2 out]
            n151 = property on="CH 9 FAIL" class="Bool (strict)"("Value"=w318) -> ()  [unwired: 2 in, 2 out]
          }
          frame 4 {
          }
        }
        n152 = case "Channel 10" shown="2" w277 {
          tunnel: ["Part Connected" "Part Connected" w304 "IDLE" "Part Connected"] -> w285
          tunnel: w270 -> [_ _ w303 _ _]
          frame 0, Default {
          }
          frame 1 {
          }
          frame 2 {
            n153 = case shown="False" w303 {
              tunnel: ["Old Part" "Retest"] -> w304
              frame False {
              }
              frame True {
              }
            }
          }
          frame 3 {
            w308 = FALSE
            n154 = property on="CH 10 RES VAL" class="Str"("Value"="") -> ()  [unwired: 2 in, 2 out]
            n155 = property on="CH 10  PASS" class="Bool (strict)"("Value"=w308) -> ()  [unwired: 2 in, 2 out]
            n156 = property on="CH 10 FAIL" class="Bool (strict)"("Value"=w308) -> ()  [unwired: 2 in, 2 out]
          }
          frame 4 {
          }
        }
        n157 = case "Channel 1" shown="2" w295 {
          tunnel: ["Part Connected" "Part Connected" w394 "IDLE" "Part Connected"] -> w294
          tunnel: w270 -> [_ _ w393 _ _]
          frame 0, Default {
          }
          frame 1 {
          }
          frame 2 {
            n158 = case shown="False" w393 {
              tunnel: ["Old Part" "Retest"] -> w394
              frame False {
              }
              frame True {
              }
            }
          }
          frame 3 {
            w398 = FALSE
            n159 = property on="CH 1 RES VAL" class="Str"("Value"="") -> ()  [unwired: 2 in, 2 out]
            n160 = property on="CH 1 PASS" class="Bool (strict)"("Value"=w398) -> ()  [unwired: 2 in, 2 out]
            n161 = property on="CH 1 FAIL" class="Bool (strict)"("Value"=w398) -> ()  [unwired: 2 in, 2 out]
          }
          frame 4 {
          }
        }
        n162 = case "Channel 2" shown="3" w284 {
          tunnel: ["Part Connected" "Part Connected" w384 "IDLE" "Part Connected"] -> w293
          tunnel: w270 -> [_ _ w383 _ _]
          frame 0, Default {
          }
          frame 1 {
          }
          frame 2 {
            n163 = case shown="False" w383 {
              tunnel: ["Old Part" "Retest"] -> w384
              frame False {
              }
              frame True {
              }
            }
          }
          frame 3 {
            w388 = FALSE
            n164 = property on="CH 2 RES VAL" class="Str"("Value"="") -> ()  [unwired: 2 in, 2 out]
            n165 = property on="CH 2 PASS" class="Bool (strict)"("Value"=w388) -> ()  [unwired: 2 in, 2 out]
            n166 = property on="CH 2 FAIL" class="Bool (strict)"("Value"=w388) -> ()  [unwired: 2 in, 2 out]
          }
          frame 4 {
          }
        }
        n167 = case "Channel 3" shown="2" w283 {
          tunnel: ["Partr Connected" "Part Connected" w374 "IDLE" "Part Connected"] -> w292
          tunnel: w270 -> [_ _ w373 _ _]
          frame 0, Default {
          }
          frame 1 {
          }
          frame 2 {
            n168 = case shown="False" w373 {
              tunnel: ["Old Part" "Retest"] -> w374
              frame False {
              }
              frame True {
              }
            }
          }
          frame 3 {
            w378 = FALSE
            n169 = property on="CH 3 RES VAL" class="Str"("Value"="") -> ()  [unwired: 2 in, 2 out]
            n170 = property on="CH 3 PASS" class="Bool (strict)"("Value"=w378) -> ()  [unwired: 2 in, 2 out]
            n171 = property on="CH 3 FAIL" class="Bool (strict)"("Value"=w378) -> ()  [unwired: 2 in, 2 out]
          }
          frame 4 {
          }
        }
        n172 = case "Channel 4" shown="2" w282 {
          tunnel: ["Part Connected" "Part Connected" w364 "IDLE" "Part Connected"] -> w291
          tunnel: w270 -> [_ _ w363 _ _]
          frame 0, Default {
          }
          frame 1 {
          }
          frame 2 {
            n173 = case shown="False" w363 {
              tunnel: ["Old Part" "Retest"] -> w364
              frame False {
              }
              frame True {
              }
            }
          }
          frame 3 {
            w368 = FALSE
            n174 = property on="CH 4 RES VAL" class="Str"("Value"="") -> ()  [unwired: 2 in, 2 out]
            n175 = property on="CH 4 PASS" class="Bool (strict)"("Value"=w368) -> ()  [unwired: 2 in, 2 out]
            n176 = property on="CH 4 FAIL" class="Bool (strict)"("Value"=w368) -> ()  [unwired: 2 in, 2 out]
          }
          frame 4 {
          }
        }
        n177 = case "Channel 5" shown="2" w269 {
          tunnel: ["Part Connected" "Part Connected" w354 "IDLE" "Part Connected"] -> w290
          tunnel: w270 -> [_ _ w353 _ _]
          frame 0, Default {
          }
          frame 1 {
          }
          frame 2 {
            n178 = case shown="False" w353 {
              tunnel: ["Old Part" "Retest"] -> w354
              frame False {
              }
              frame True {
              }
            }
          }
          frame 3 {
            w358 = FALSE
            n179 = property on="CH 5 RES VAL" class="Str"("Value"="") -> ()  [unwired: 2 in, 2 out]
            n180 = property on="CH 5 PASS" class="Bool (strict)"("Value"=w358) -> ()  [unwired: 2 in, 2 out]
            n181 = property on="CH 5 FAIL" class="Bool (strict)"("Value"=w358) -> ()  [unwired: 2 in, 2 out]
          }
          frame 4 {
          }
        }
        n182 = case "Channel 6" shown="2" w281 {
          tunnel: ["Part Connected" "Part Connected" "Part Connected" w345 "IDLE"] -> w289
          tunnel: w270 -> [_ _ _ w344 _]
          frame 0, Default {
          }
          frame 4 {
          }
          frame 1 {
          }
          frame 2 {
            n183 = case shown="False" w344 {
              tunnel: ["Old Part" "Retest"] -> w345
              frame False {
              }
              frame True {
              }
            }
          }
          frame 3 {
            w349 = FALSE
            n184 = property on="CH 6 RES VAL" class="Str"("Value"="") -> ()  [unwired: 2 in, 2 out]
            n185 = property on="CH 6 PASS" class="Bool (strict)"("Value"=w349) -> ()  [unwired: 2 in, 2 out]
            n186 = property on="CH 6 FAIL" class="Bool (strict)"("Value"=w349) -> ()  [unwired: 2 in, 2 out]
          }
        }
        n187 = case "Channel 7" shown="2" w280 {
          tunnel: ["Part Connected" "Part Connected" w334 "IDLE" "Part Connected"] -> w288
          tunnel: w270 -> [_ _ w333 _ _]
          frame 0, Default {
          }
          frame 1 {
          }
          frame 2 {
            n188 = case shown="True" w333 {
              tunnel: ["Old Part" "Retest"] -> w334
              frame False {
              }
              frame True {
              }
            }
          }
          frame 3 {
            w338 = FALSE
            n189 = property on="CH 7 RES VAL" class="Str"("Value"="") -> ()  [unwired: 2 in, 2 out]
            n190 = property on="CH 7 PASS" class="Bool (strict)"("Value"=w338) -> ()  [unwired: 2 in, 2 out]
            n191 = property on="CH 7 FAIL" class="Bool (strict)"("Value"=w338) -> ()  [unwired: 2 in, 2 out]
          }
          frame 4 {
          }
        }
        n192 = property on="CH 8 STATUS" class="Str"("Value"=w287) -> ()  [unwired: 2 in, 2 out]
        n193 = property on="CH 9 STATUS" class="Str"("Value"=w286) -> ()  [unwired: 2 in, 2 out]
        n194 = property on="CH 10 STATUS" class="Str"("Value"=w285) -> ()  [unwired: 2 in, 2 out]
        n195 = property on="CH1 STATUS" class="Str"("Value"=w294) -> ()  [unwired: 2 in, 2 out]
        n196 = property on="CH 2 STATUS" class="Str"("Value"=w293) -> ()  [unwired: 2 in, 2 out]
        n197 = property on="CH 4 STATUS" class="Str"("Value"=w291) -> ()  [unwired: 2 in, 2 out]
        n198 = property on="CH 5 STATUS" class="Str"("Value"=w290) -> ()  [unwired: 2 in, 2 out]
        n199 = property on="CH 6 STATUS" class="Str"("Value"=w289) -> ()  [unwired: 2 in, 2 out]
        n200 = property on="CH 7 STATUS" class="Str"("Value"=w288) -> ()  [unwired: 2 in, 2 out]
        n201 = property on="CH 3 STATUS" class="Str"("Value"=w292) -> ()  [unwired: 2 in, 2 out]
        n202 = case shown="9" w268 {
          tunnel: [TEST_ENNUM."TIMEOUT" TEST_ENNUM."TIMEOUT" TEST_ENNUM."VALIDATING"] -> w267
          frame 8, Default {
          }
          frame 6 {
            n203 = One Button Dialog(message="NO PART IN REFERENCE CHANNEL", button name ("OK")="OK") -> ()  [unwired: 1 out]
          }
          frame 9 {
          }
        }
      }
      frame "VALIDATING" {
        n204 = Unbundle By Name(w423) -> ("MODE"=w538:string, "RES VALUE 5"=w421:dbl)
        n205 = Equal?(x=w538, y="USER MODE") -> (x = y?=w424:bool)
        n206 = case shown="False" w424 {
          tunnel: [w540 w542] -> w422
          tunnel: w423 -> [w541 w542]
          tunnel: w421 -> [w539 _]
          frame False {
            n207 = Bundle By Name(cluster=w541, "SET VALUE 1"=w539, "SET VALUE 2"=w539, "SET VALUE 3"=w539, "SET VALUE 4"=w539, "SET VALUE 5"=w539, "SET VALUE 6"=w539, "SET VALUE 7"=w539, "SET VALUE 8"=w539, "SET VALUE 9"=w539, "SET VALUE 10"=w539) -> (w540:T2)
          }
          frame True {
          }
        }
        n208 = Unbundle By Name(w422) -> ("PP 1"=w533:i32, "PP 2"=w515:i32, "PP 3"=w514:i32, "PP 4"=w513:i32, "PP 5"=w512:i32, "PP 6"=w511:i32, "PP 7"=w510:i32, "PP 8"=w509:i32, "PP 9"=w508:i32, "PP 10"=w505:i32)
        n209 = Equal?(x=w533, y=2) -> (x = y?=w503:bool)
        n210 = Equal?(x=w533, y=1) -> (x = y?=w502:bool)
        n211 = Equal?(x=w515, y=2) -> (x = y?=w496:bool)
        n212 = Equal?(x=w515, y=1) -> (x = y?=w495:bool)
        n213 = Equal?(x=w514, y=2) -> (x = y?=w494:bool)
        n214 = Equal?(x=w514, y=1) -> (x = y?=w493:bool)
        n215 = Equal?(x=w513, y=2) -> (x = y?=w488:bool)
        n216 = Equal?(x=w513, y=1) -> (x = y?=w489:bool)
        n217 = Equal?(x=w512, y=2) -> (x = y?=w482:bool)
        n218 = Equal?(x=w512, y=1) -> (x = y?=w483:bool)
        n219 = Equal?(x=w511, y=2) -> (x = y?=w479:bool)
        n220 = Equal?(x=w511, y=1) -> (x = y?=w480:bool)
        n221 = Equal?(x=w510, y=2) -> (x = y?=w475:bool)
        n222 = Equal?(x=w510, y=1) -> (x = y?=w474:bool)
        n223 = Equal?(x=w509, y=2) -> (x = y?=w470:bool)
        n224 = Equal?(x=w509, y=1) -> (x = y?=w469:bool)
        n225 = Equal?(x=w508, y=2) -> (x = y?=w465:bool)
        n226 = Equal?(x=w505, y=2) -> (x = y?=w462:bool)
        n227 = Equal?(x=w508, y=1) -> (x = y?=w463:bool)
        n228 = Equal?(x=w505, y=1) -> (x = y?=w464:bool)
        n229 = Or(x=w488, y=w489) -> (x .or. y?=w487:bool)
        n230 = Or(x=w482, y=w483) -> (x .or. y?=w481:bool)
        n231 = Or(x=w479, y=w480) -> (x .or. y?=w478:bool)
        n232 = Or(x=w503, y=w502) -> (x .or. y?=w504:bool)
        n233 = Or(x=w496, y=w495) -> (x .or. y?=w497:bool)
        n234 = Or(x=w494, y=w493) -> (x .or. y?=w492:bool)
        n235 = Or(x=w475, y=w474) -> (x .or. y?=w471:bool)
        n236 = Or(x=w470, y=w469) -> (x .or. y?=w468:bool)
        n237 = Or(x=w465, y=w463) -> (x .or. y?=w461:bool)
        n238 = Or(x=w462, y=w464) -> (x .or. y?=w460:bool)
        n239 = Unbundle By Name(w422) -> ("SET VALUE 1"=w501:dbl, "SET VALUE 2"=w500:dbl, "SET VALUE 3"=w491:dbl, "SET VALUE 4"=w486:dbl, "SET VALUE 5"=w484:dbl, "SET VALUE 6"=w473:dbl, "SET VALUE 7"=w435:dbl, "SET VALUE 8"=w467:dbl, "SET VALUE 9"=w459:dbl, "SET VALUE 10"=w457:dbl, "TOL 1"=w499:dbl, "TOL 2"=w498:dbl, "TOL 3"=w490:dbl, "TOL 4"=w485:dbl, "TOL 5"=w477:dbl, "TOL 6"=w476:dbl, "TOL 7"=w472:dbl, "TOL 8"=w466:dbl, "TOL 9"=w458:dbl, "TOL 10"=w456:dbl, "RES VALUE 1"=w434:dbl, "RES VALUE 2"=w433:dbl, "RES VALUE 3"=w432:dbl, "RES VALUE 4"=w431:dbl, "RES VALUE 5"=w430:dbl, "RES VALUE 6"=w429:dbl, "RES VALUE 7"=w428:dbl, "RES VALUE 8"=w427:dbl, "RES VALUE 9"=w426:dbl, "RES VALUE 10"=w425:dbl)
        n240 = case "Channel 1" shown="True" w504 {
          tunnel: w501 -> [_ w639]
          tunnel: w499 -> [_ w640]
          tunnel: [_ w637] -> w455
          tunnel: [_ w636] -> w454
          tunnel: w434 -> [_ w635]
          tunnel: [_ w634] -> w420
          tunnel: [_ w633] -> w419
          frame False {
          }
          frame True {
            n241 = call "TOL_EQ.vi"("TOL VALUE"=w640, "NOM VALUE"=w639) -> ("MIN"=w633:dbl, "MAX"=w634:dbl)  [unwired: 8 in]
            n242 = In Range and Coerce(upper limit=w634, x=w635, lower limit=w633) -> (In Range?=w638:bool)  [unwired: 1 out]
            n243 = case shown="False" w638 {
              tunnel: [_ TRUE] -> w637
              tunnel: [TRUE _] -> w636
              frame False {
              }
              frame True {
              }
            }
          }
        }
        n244 = case "Channel 2" shown="True" w497 {
          tunnel: w500 -> [_ w629]
          tunnel: w498 -> [_ w630]
          tunnel: [_ w627] -> w453
          tunnel: [_ w626] -> w452
          tunnel: w433 -> [_ w625]
          tunnel: [_ w624] -> w418
          tunnel: [_ w623] -> w417
          frame False {
          }
          frame True {
            n245 = call "TOL_EQ.vi"("TOL VALUE"=w630, "NOM VALUE"=w629) -> ("MIN"=w623:dbl, "MAX"=w624:dbl)  [unwired: 8 in]
            n246 = In Range and Coerce(upper limit=w624, x=w625, lower limit=w623) -> (In Range?=w628:bool)  [unwired: 1 out]
            n247 = case shown="False" w628 {
              tunnel: [_ TRUE] -> w627
              tunnel: [TRUE _] -> w626
              frame False {
              }
              frame True {
              }
            }
          }
        }
        n248 = case "Channel 3" shown="True" w492 {
          tunnel: w491 -> [_ w619]
          tunnel: w490 -> [_ w620]
          tunnel: [_ w617] -> w451
          tunnel: [_ w616] -> w450
          tunnel: w432 -> [_ w615]
          tunnel: [_ w614] -> w416
          tunnel: [_ w613] -> w415
          frame False {
          }
          frame True {
            n249 = call "TOL_EQ.vi"("TOL VALUE"=w620, "NOM VALUE"=w619) -> ("MIN"=w613:dbl, "MAX"=w614:dbl)  [unwired: 8 in]
            n250 = In Range and Coerce(upper limit=w614, x=w615, lower limit=w613) -> (In Range?=w618:bool)  [unwired: 1 out]
            n251 = case shown="True" w618 {
              tunnel: [_ TRUE] -> w617
              tunnel: [TRUE _] -> w616
              frame False {
              }
              frame True {
              }
            }
          }
        }
        n252 = case "Channel 4" shown="True" w487 {
          tunnel: w486 -> [_ w609]
          tunnel: w485 -> [_ w610]
          tunnel: [_ w607] -> w449
          tunnel: [_ w606] -> w448
          tunnel: w431 -> [_ w605]
          tunnel: [_ w604] -> w414
          tunnel: [_ w603] -> w413
          frame False {
          }
          frame True {
            n253 = call "TOL_EQ.vi"("TOL VALUE"=w610, "NOM VALUE"=w609) -> ("MIN"=w603:dbl, "MAX"=w604:dbl)  [unwired: 8 in]
            n254 = In Range and Coerce(upper limit=w604, x=w605, lower limit=w603) -> (In Range?=w608:bool)  [unwired: 1 out]
            n255 = case shown="False" w608 {
              tunnel: [_ TRUE] -> w607
              tunnel: [TRUE _] -> w606
              frame False {
              }
              frame True {
              }
            }
          }
        }
        n256 = case "Channel 5" shown="False" w481 {
          tunnel: w484 -> [_ w599]
          tunnel: w477 -> [_ w600]
          tunnel: [_ w597] -> w447
          tunnel: [_ w596] -> w446
          tunnel: w430 -> [_ w595]
          tunnel: [_ w594] -> w412
          tunnel: [_ w593] -> w411
          frame False {
          }
          frame True {
            n257 = call "TOL_EQ.vi"("TOL VALUE"=w600, "NOM VALUE"=w599) -> ("MIN"=w593:dbl, "MAX"=w594:dbl)  [unwired: 8 in]
            n258 = In Range and Coerce(upper limit=w594, x=w595, lower limit=w593) -> (In Range?=w598:bool)  [unwired: 1 out]
            n259 = case shown="False" w598 {
              tunnel: [_ TRUE] -> w597
              tunnel: [TRUE _] -> w596
              frame False {
              }
              frame True {
              }
            }
          }
        }
        n260 = case "Channel 6" shown="False" w478 {
          tunnel: w473 -> [_ w589]
          tunnel: w476 -> [_ w590]
          tunnel: [_ w587] -> w445
          tunnel: [_ w586] -> w444
          tunnel: w429 -> [_ w585]
          tunnel: [_ w584] -> w410
          tunnel: [_ w583] -> w409
          frame False {
          }
          frame True {
            n261 = call "TOL_EQ.vi"("TOL VALUE"=w590, "NOM VALUE"=w589) -> ("MIN"=w583:dbl, "MAX"=w584:dbl)  [unwired: 8 in]
            n262 = In Range and Coerce(upper limit=w584, x=w585, lower limit=w583) -> (In Range?=w588:bool)  [unwired: 1 out]
            n263 = case shown="False" w588 {
              tunnel: [_ TRUE] -> w587
              tunnel: [TRUE _] -> w586
              frame False {
              }
              frame True {
              }
            }
          }
        }
        n264 = case "Channel 10" shown="False" w460 {
          tunnel: w457 -> [_ w549]
          tunnel: w456 -> [_ w550]
          tunnel: [_ w547] -> w437
          tunnel: [_ w546] -> w436
          tunnel: w425 -> [_ w545]
          tunnel: [_ w544] -> w402
          tunnel: [_ w543] -> w401
          frame False {
          }
          frame True {
            n265 = call "TOL_EQ.vi"("TOL VALUE"=w550, "NOM VALUE"=w549) -> ("MIN"=w543:dbl, "MAX"=w544:dbl)  [unwired: 8 in]
            n266 = In Range and Coerce(upper limit=w544, x=w545, lower limit=w543) -> (In Range?=w548:bool)  [unwired: 1 out]
            n267 = case shown="False" w548 {
              tunnel: [_ TRUE] -> w547
              tunnel: [TRUE _] -> w546
              frame False {
              }
              frame True {
              }
            }
          }
        }
        n268 = case "Channel 7" shown="False" w471 {
          tunnel: w472 -> [_ w580]
          tunnel: [_ w578] -> w443
          tunnel: [_ w577] -> w442
          tunnel: w435 -> [_ w576]
          tunnel: w428 -> [_ w575]
          tunnel: [_ w574] -> w408
          tunnel: [_ w573] -> w407
          frame False {
          }
          frame True {
            n269 = call "TOL_EQ.vi"("TOL VALUE"=w580, "NOM VALUE"=w576) -> ("MIN"=w573:dbl, "MAX"=w574:dbl)  [unwired: 8 in]
            n270 = In Range and Coerce(upper limit=w574, x=w575, lower limit=w573) -> (In Range?=w579:bool)  [unwired: 1 out]
            n271 = case shown="False" w579 {
              tunnel: [_ TRUE] -> w578
              tunnel: [TRUE _] -> w577
              frame False {
              }
              frame True {
              }
            }
          }
        }
        n272 = case "Channel 8" shown="True" w468 {
          tunnel: w467 -> [_ w569]
          tunnel: w466 -> [_ w570]
          tunnel: [_ w567] -> w441
          tunnel: [_ w566] -> w440
          tunnel: w427 -> [_ w565]
          tunnel: [_ w564] -> w406
          tunnel: [_ w563] -> w405
          frame False {
          }
          frame True {
            n273 = call "TOL_EQ.vi"("TOL VALUE"=w570, "NOM VALUE"=w569) -> ("MIN"=w563:dbl, "MAX"=w564:dbl)  [unwired: 8 in]
            n274 = In Range and Coerce(upper limit=w564, x=w565, lower limit=w563) -> (In Range?=w568:bool)  [unwired: 1 out]
            n275 = case shown="False" w568 {
              tunnel: [_ TRUE] -> w567
              tunnel: [TRUE _] -> w566
              frame False {
              }
              frame True {
              }
            }
          }
        }
        n276 = case "Channel 9" shown="False" w461 {
          tunnel: w459 -> [_ w559]
          tunnel: w458 -> [_ w560]
          tunnel: [_ w557] -> w439
          tunnel: [_ w556] -> w438
          tunnel: w426 -> [_ w555]
          tunnel: [_ w554] -> w404
          tunnel: [_ w553] -> w403
          frame False {
          }
          frame True {
            n277 = call "TOL_EQ.vi"("TOL VALUE"=w560, "NOM VALUE"=w559) -> ("MIN"=w553:dbl, "MAX"=w554:dbl)  [unwired: 8 in]
            n278 = In Range and Coerce(upper limit=w554, x=w555, lower limit=w553) -> (In Range?=w558:bool)  [unwired: 1 out]
            n279 = case shown="False" w558 {
              tunnel: [_ TRUE] -> w557
              tunnel: [TRUE _] -> w556
              frame False {
              }
              frame True {
              }
            }
          }
        }
        n280 = Bundle By Name(cluster=w422, "CH  PASS  1"=w455, "CH  PASS 2"=w453, "CH  PASS 3"=w451, "CH  PASS 4"=w449, "CH  PASS 5"=w447, "CH  PASS 6"=w445, "CH  PASS 7"=w443, "CH  PASS 8"=w441, "CH  PASS 9"=w439, "CH  PASS 10"=w437, "CH  FAIL 1"=w454, "CH  FAIL 2"=w452, "CH  FAIL 3"=w450, "CH  FAIL 4"=w448, "CH  FAIL 5"=w446, "CH  FAIL 6"=w444, "CH  FAIL 7"=w442, "CH  FAIL 8"=w440, "CH  FAIL 9"=w438, "CH  FAIL 10"=w436, "CH1 MIN TOL"=w419, "CH2 MIN TOL"=w417, "CH3 MIN TOL"=w415, "CH4 MIN TOL"=w413, "CH5 MIN TOL"=w411, "CH6 MIN TOL"=w409, "CH7 MIN TOL"=w407, "CH8 MIN TOL"=w405, "CH9 MIN TOL"=w403, "CH10 MIN TOL"=w401, "CH1 MAX TOL"=w420, "CH2 MAX TOL"=w418, "CH3 MAX TOL"=w416, "CH4 MAX TOL"=w414, "CH5 MAX TOL"=w412, "CH6 MAX TOL"=w410, "CH7 MAX TOL"=w408, "CH8 MAX TOL"=w406, "CH9 MAX TOL"=w404, "CH10 MAX TOL"=w402) -> (w536:T2)
      }
      frame "RESULT" {
        n281 = Unbundle By Name(w643) -> ("PP 1"=w679:i32, "PP 2"=w676:i32, "PP 3"=w673:i32, "PP 4"=w670:i32, "PP 5"=w667:i32, "PP 6"=w664:i32, "PP 7"=w661:i32, "PP 8"=w658:i32, "PP 9"=w655:i32, "PP 10"=w652:i32, "CH  PASS  1"=w678:bool, "CH  PASS 2"=w675:bool, "CH  PASS 3"=w672:bool, "CH  PASS 4"=w669:bool, "CH  PASS 5"=w666:bool, "CH  PASS 6"=w663:bool, "CH  PASS 7"=w660:bool, "CH  PASS 8"=w657:bool, "CH  PASS 9"=w654:bool, "CH  PASS 10"=w651:bool, "CH  FAIL 1"=w677:bool, "CH  FAIL 2"=w674:bool, "CH  FAIL 3"=w671:bool, "CH  FAIL 4"=w668:bool, "CH  FAIL 5"=w665:bool, "CH  FAIL 6"=w662:bool, "CH  FAIL 7"=w659:bool, "CH  FAIL 8"=w656:bool, "CH  FAIL 9"=w653:bool, "CH  FAIL 10"=w650:bool, "RES VALUE 1"=w646:dbl, "RES VALUE 2"=w704:dbl, "RES VALUE 3"=w703:dbl, "RES VALUE 4"=w702:dbl, "RES VALUE 5"=w701:dbl, "RES VALUE 6"=w700:dbl, "RES VALUE 7"=w649:dbl, "RES VALUE 8"=w699:dbl, "RES VALUE 9"=w698:dbl, "RES VALUE 10"=w697:dbl, "PP 1"=w647:i32, "PP 2"=w687:i32, "PP 3"=w686:i32, "PP 4"=w685:i32, "PP 5"=w684:i32, "PP 6"=w683:i32, "PP 7"=w648:i32, "PP 8"=w682:i32, "PP 9"=w681:i32, "PP 10"=w680:i32)
        n282 = case shown="2" w679 {
          tunnel: w678 -> [_ w752 w754]
          tunnel: w677 -> [_ w751 w753]
          frame 0, Default {
          }
          frame 1 {
            n283 = property on="CH 1 PASS" class="Bool (strict)"("Value"=w752) -> ()  [unwired: 2 in, 2 out]
            n284 = property on="CH 1 FAIL" class="Bool (strict)"("Value"=w751) -> ()  [unwired: 2 in, 2 out]
          }
          frame 2 {
            n285 = property on="CH 1 FAIL" class="Bool (strict)"("Value"=w753) -> ()  [unwired: 2 in, 2 out]
            n286 = property on="CH 1 PASS" class="Bool (strict)"("Value"=w754) -> ()  [unwired: 2 in, 2 out]
          }
        }
        n287 = case shown="3" w647 {
          tunnel: w646 -> [_ w707 w711 _]
          tunnel: ["0" w706 w710 ""] -> w645
          frame 0, Default {
          }
          frame 1 {
            n288 = Number To Fractional String(use system decimal point (T)=TRUE, number=w707, precision (6)=i16 3) -> (F-format string=w706:string)  [unwired: 1 in]
          }
          frame 2 {
            n289 = Number To Fractional String(use system decimal point (T)=TRUE, number=w711, precision (6)=i16 3) -> (F-format string=w710:string)  [unwired: 1 in]
          }
          frame 3 {
          }
        }
        n290 = case shown="3" w687 {
          tunnel: w704 -> [_ w836 w840 _]
          tunnel: ["0" w835 w839 ""] -> w696
          frame 0, Default {
          }
          frame 1 {
            n291 = Number To Fractional String(use system decimal point (T)=TRUE, number=w836, precision (6)=i16 3) -> (F-format string=w835:string)  [unwired: 1 in]
          }
          frame 2 {
            n292 = Number To Fractional String(use system decimal point (T)=TRUE, number=w840, precision (6)=i16 3) -> (F-format string=w839:string)  [unwired: 1 in]
          }
          frame 3 {
          }
        }
        n293 = case shown="0, Default" w686 {
          tunnel: w703 -> [_ w827 w831 _]
          tunnel: ["" w826 w830 _] -> w695
          frame 0, Default {
          }
          frame 1 {
            n294 = Number To Fractional String(use system decimal point (T)=TRUE, number=w827, precision (6)=i16 3) -> (F-format string=w826:string)  [unwired: 1 in]
          }
          frame 2 {
            n295 = Number To Fractional String(use system decimal point (T)=TRUE, number=w831, precision (6)=i16 3) -> (F-format string=w830:string)  [unwired: 1 in]
          }
          frame 3 {
          }
        }
        n296 = case shown="3" w685 {
          tunnel: w702 -> [_ w817 w821 _]
          tunnel: ["0" w816 w820 ""] -> w694
          frame 0, Default {
          }
          frame 1 {
            n297 = Number To Fractional String(use system decimal point (T)=TRUE, number=w817, precision (6)=i16 3) -> (F-format string=w816:string)  [unwired: 1 in]
          }
          frame 2 {
            n298 = Number To Fractional String(use system decimal point (T)=TRUE, number=w821, precision (6)=i16 3) -> (F-format string=w820:string)  [unwired: 1 in]
          }
          frame 3 {
          }
        }
        n299 = case shown="3" w684 {
          tunnel: w701 -> [_ w807 w810 _]
          tunnel: ["0" w806 w811 ""] -> w693
          frame 0, Default {
          }
          frame 1 {
            n300 = Number To Fractional String(use system decimal point (T)=TRUE, number=w807, precision (6)=i16 3) -> (F-format string=w806:string)  [unwired: 1 in]
          }
          frame 2 {
            n301 = Number To Fractional String(use system decimal point (T)=TRUE, number=w810, precision (6)=i16 3) -> (F-format string=w811:string)  [unwired: 1 in]
          }
          frame 3 {
          }
        }
        n302 = case shown="3" w683 {
          tunnel: w700 -> [_ w797 w801 _]
          tunnel: ["0" w796 w800 ""] -> w692
          frame 0, Default {
          }
          frame 1 {
            n303 = Number To Fractional String(use system decimal point (T)=TRUE, number=w797, precision (6)=i16 3) -> (F-format string=w796:string)  [unwired: 1 in]
          }
          frame 2 {
            n304 = Number To Fractional String(use system decimal point (T)=TRUE, number=w801, precision (6)=i16 3) -> (F-format string=w800:string)  [unwired: 1 in]
          }
          frame 3 {
          }
        }
        n305 = case shown="3" w648 {
          tunnel: w649 -> [_ w787 w791 _]
          tunnel: ["0" w786 w790 ""] -> w691
          frame 0, Default {
          }
          frame 1 {
            n306 = Number To Fractional String(use system decimal point (T)=TRUE, number=w787, precision (6)=i16 3) -> (F-format string=w786:string)  [unwired: 1 in]
          }
          frame 2 {
            n307 = Number To Fractional String(use system decimal point (T)=TRUE, number=w791, precision (6)=i16 3) -> (F-format string=w790:string)  [unwired: 1 in]
          }
          frame 3 {
          }
        }
        n308 = case shown="3" w682 {
          tunnel: w699 -> [_ w777 w781 _]
          tunnel: ["0" w776 w780 ""] -> w690
          frame 0, Default {
          }
          frame 1 {
            n309 = Number To Fractional String(use system decimal point (T)=TRUE, number=w777, precision (6)=i16 3) -> (F-format string=w776:string)  [unwired: 1 in]
          }
          frame 2 {
            n310 = Number To Fractional String(use system decimal point (T)=TRUE, number=w781, precision (6)=i16 3) -> (F-format string=w780:string)  [unwired: 1 in]
          }
          frame 3 {
          }
        }
        n311 = case shown="3" w681 {
          tunnel: w698 -> [_ w767 w771 _]
          tunnel: ["" w766 w770 ""] -> w689
          frame 0, Default {
          }
          frame 1 {
            n312 = Number To Fractional String(use system decimal point (T)=TRUE, number=w767, precision (6)=i16 3) -> (F-format string=w766:string)  [unwired: 1 in]
          }
          frame 2 {
            n313 = Number To Fractional String(use system decimal point (T)=TRUE, number=w771, precision (6)=i16 3) -> (F-format string=w770:string)  [unwired: 1 in]
          }
          frame 3 {
          }
        }
        n314 = case shown="3" w680 {
          tunnel: w697 -> [_ w759 w761 _]
          tunnel: ["0" w758 w760 ""] -> w688
          frame 0, Default {
          }
          frame 1 {
            n315 = Number To Fractional String(use system decimal point (T)=TRUE, number=w759, precision (6)=i16 3) -> (F-format string=w758:string)  [unwired: 1 in]
          }
          frame 2 {
            n316 = Number To Fractional String(use system decimal point (T)=TRUE, number=w761, precision (6)=i16 3) -> (F-format string=w760:string)  [unwired: 1 in]
          }
          frame 3 {
          }
        }
        n317 = property on="CH 1 RES VAL" class="Str"("Value"=w645) -> ()  [unwired: 2 in, 2 out]
        n318 = property on="CH 2 RES VAL" class="Str"("Value"=w696) -> ()  [unwired: 2 in, 2 out]
        n319 = property on="CH 3 RES VAL" class="Str"("Value"=w695) -> ()  [unwired: 2 in, 2 out]
        n320 = property on="CH 4 RES VAL" class="Str"("Value"=w694) -> ()  [unwired: 2 in, 2 out]
        n321 = property on="CH 5 RES VAL" class="Str"("Value"=w693) -> ()  [unwired: 2 in, 2 out]
        n322 = property on="CH 6 RES VAL" class="Str"("Value"=w692) -> ()  [unwired: 2 in, 2 out]
        n323 = property on="CH 7 RES VAL" class="Str"("Value"=w691) -> ()  [unwired: 2 in, 2 out]
        n324 = property on="CH 8 RES VAL" class="Str"("Value"=w690) -> ()  [unwired: 2 in, 2 out]
        n325 = property on="CH 9 RES VAL" class="Str"("Value"=w689) -> ()  [unwired: 2 in, 2 out]
        n326 = property on="CH 10 RES VAL" class="Str"("Value"=w688) -> ()  [unwired: 2 in, 2 out]
        n327 = case shown="2" w676 {
          tunnel: w675 -> [_ w748 w750 _]
          tunnel: w674 -> [_ w747 w749 _]
          frame 0, Default {
          }
          frame 1 {
            n328 = property on="CH 2 PASS" class="Bool (strict)"("Value"=w748) -> ()  [unwired: 2 in, 2 out]
            n329 = property on="CH 2 FAIL" class="Bool (strict)"("Value"=w747) -> ()  [unwired: 2 in, 2 out]
          }
          frame 2 {
            n330 = property on="CH 2 PASS" class="Bool (strict)"("Value"=w750) -> ()  [unwired: 2 in, 2 out]
            n331 = property on="CH 2 FAIL" class="Bool (strict)"("Value"=w749) -> ()  [unwired: 2 in, 2 out]
          }
          frame 3 {
          }
        }
        n332 = case shown="1" w673 {
          tunnel: w672 -> [_ w744 w746 _]
          tunnel: w671 -> [_ w743 w745 _]
          frame 0, Default {
          }
          frame 1 {
            n333 = property on="CH 3 PASS" class="Bool (strict)"("Value"=w744) -> ()  [unwired: 2 in, 2 out]
            n334 = property on="CH 3 FAIL" class="Bool (strict)"("Value"=w743) -> ()  [unwired: 2 in, 2 out]
          }
          frame 2 {
            n335 = property on="CH 3 PASS" class="Bool (strict)"("Value"=w746) -> ()  [unwired: 2 in, 2 out]
            n336 = property on="CH 3 FAIL" class="Bool (strict)"("Value"=w745) -> ()  [unwired: 2 in, 2 out]
          }
          frame 3 {
          }
        }
        n337 = case shown="1" w670 {
          tunnel: w669 -> [_ w740 w742 _]
          tunnel: w668 -> [_ w739 w741 _]
          frame 0, Default {
          }
          frame 1 {
            n338 = property on="CH 4 PASS" class="Bool (strict)"("Value"=w740) -> ()  [unwired: 2 in, 2 out]
            n339 = property on="CH 4 FAIL" class="Bool (strict)"("Value"=w739) -> ()  [unwired: 2 in, 2 out]
          }
          frame 2 {
            n340 = property on="CH 4 PASS" class="Bool (strict)"("Value"=w742) -> ()  [unwired: 2 in, 2 out]
            n341 = property on="CH 4 FAIL" class="Bool (strict)"("Value"=w741) -> ()  [unwired: 2 in, 2 out]
          }
          frame 3 {
          }
        }
        n342 = case shown="1" w667 {
          tunnel: w666 -> [_ w736 w738 _]
          tunnel: w665 -> [_ w735 w737 _]
          frame 0, Default {
          }
          frame 1 {
            n343 = property on="CH 5 PASS" class="Bool (strict)"("Value"=w736) -> ()  [unwired: 2 in, 2 out]
            n344 = property on="CH 5 FAIL" class="Bool (strict)"("Value"=w735) -> ()  [unwired: 2 in, 2 out]
          }
          frame 2 {
            n345 = property on="CH 5 PASS" class="Bool (strict)"("Value"=w738) -> ()  [unwired: 2 in, 2 out]
            n346 = property on="CH 5 FAIL" class="Bool (strict)"("Value"=w737) -> ()  [unwired: 2 in, 2 out]
          }
          frame 3 {
          }
        }
        n347 = case shown="1" w664 {
          tunnel: w663 -> [_ w732 w734 _]
          tunnel: w662 -> [_ w731 w733 _]
          frame 0, Default {
          }
          frame 1 {
            n348 = property on="CH 6 PASS" class="Bool (strict)"("Value"=w732) -> ()  [unwired: 2 in, 2 out]
            n349 = property on="CH 6 FAIL" class="Bool (strict)"("Value"=w731) -> ()  [unwired: 2 in, 2 out]
          }
          frame 2 {
            n350 = property on="CH 6 FAIL" class="Bool (strict)"("Value"=w733) -> ()  [unwired: 2 in, 2 out]
            n351 = property on="CH 6 PASS" class="Bool (strict)"("Value"=w734) -> ()  [unwired: 2 in, 2 out]
          }
          frame 3 {
          }
        }
        n352 = case shown="1" w661 {
          tunnel: w660 -> [_ w728 w730 _]
          tunnel: w659 -> [_ w727 w729 _]
          frame 0, Default {
          }
          frame 1 {
            n353 = property on="CH 7 PASS" class="Bool (strict)"("Value"=w728) -> ()  [unwired: 2 in, 2 out]
            n354 = property on="CH 7 FAIL" class="Bool (strict)"("Value"=w727) -> ()  [unwired: 2 in, 2 out]
          }
          frame 2 {
            n355 = property on="CH 7 PASS" class="Bool (strict)"("Value"=w730) -> ()  [unwired: 2 in, 2 out]
            n356 = property on="CH 7 FAIL" class="Bool (strict)"("Value"=w729) -> ()  [unwired: 2 in, 2 out]
          }
          frame 3 {
          }
        }
        n357 = case shown="1" w658 {
          tunnel: w657 -> [_ w724 w726 _]
          tunnel: w656 -> [_ w723 w725 _]
          frame 0, Default {
          }
          frame 1 {
            n358 = property on="CH 8 PASS" class="Bool (strict)"("Value"=w724) -> ()  [unwired: 2 in, 2 out]
            n359 = property on="CH 8 FAIL" class="Bool (strict)"("Value"=w723) -> ()  [unwired: 2 in, 2 out]
          }
          frame 2 {
            n360 = property on="CH 8 PASS" class="Bool (strict)"("Value"=w726) -> ()  [unwired: 2 in, 2 out]
            n361 = property on="CH 8 FAIL" class="Bool (strict)"("Value"=w725) -> ()  [unwired: 2 in, 2 out]
          }
          frame 3 {
          }
        }
        n362 = case shown="1" w655 {
          tunnel: w654 -> [_ w720 w722 _]
          tunnel: w653 -> [_ w719 w721 _]
          frame 0, Default {
          }
          frame 1 {
            n363 = property on="CH 9 PASS" class="Bool (strict)"("Value"=w720) -> ()  [unwired: 2 in, 2 out]
            n364 = property on="CH 9 FAIL" class="Bool (strict)"("Value"=w719) -> ()  [unwired: 2 in, 2 out]
          }
          frame 2 {
            n365 = property on="CH 9 PASS" class="Bool (strict)"("Value"=w722) -> ()  [unwired: 2 in, 2 out]
            n366 = property on="CH 9 FAIL" class="Bool (strict)"("Value"=w721) -> ()  [unwired: 2 in, 2 out]
          }
          frame 3 {
          }
        }
        n367 = case shown="1" w652 {
          tunnel: w651 -> [_ w716 w718 _]
          tunnel: w650 -> [_ w715 w717 _]
          frame 0, Default {
          }
          frame 1 {
            n368 = property on="CH 10  PASS" class="Bool (strict)"("Value"=w716) -> ()  [unwired: 2 in, 2 out]
            n369 = property on="CH 10 FAIL" class="Bool (strict)"("Value"=w715) -> ()  [unwired: 2 in, 2 out]
          }
          frame 2 {
            n370 = property on="CH 10  PASS" class="Bool (strict)"("Value"=w718) -> ()  [unwired: 2 in, 2 out]
            n371 = property on="CH 10 FAIL" class="Bool (strict)"("Value"=w717) -> ()  [unwired: 2 in, 2 out]
          }
          frame 3 {
          }
        }
      }
      frame "LED_SEQ" {
        w859 = u16 10 items=["1.0"=10, "1.5"=15, "2.0"=20] ("stop bits (10: 1 bit)")
        w844 = 0.0 ("element")
        # "CHANNEL 9"
        # "CHANNEL 8"
        # "CHANNEL 7"
        # "CHANNEL 6"
        # "CHANNEL 5"
        # "CHANNEL 4"
        # "CHANNEL 3"
        # "CHANNEL 2"
        # "CHANNEL 1"
        n372 = Unbundle By Name(w862) -> ("VISA resource name"=w863:refnum<visa-resource-name>, "PP 1"=w892:i32, "PP 2"=w890:i32, "PP 3"=w888:i32, "PP 4"=w886:i32, "PP 5"=w884:i32, "PP 6"=w882:i32, "PP 7"=w880:i32, "PP 8"=w878:i32, "PP 9"=w876:i32, "PP 10"=w874:i32, "CH  PASS  1"=w891:bool, "CH  PASS 2"=w889:bool, "CH  PASS 3"=w887:bool, "CH  PASS 4"=w885:bool, "CH  PASS 5"=w883:bool, "CH  PASS 6"=w881:bool, "CH  PASS 7"=w879:bool, "CH  PASS 8"=w877:bool, "CH  PASS 9"=w875:bool, "CH  PASS 10"=w873:bool)
        n373 = case shown="1" w892 {
          tunnel: w891 -> [_ w1004 w1011 _]
          tunnel: [0.0 ("t") w1005 w1008 0.0 ("f")] -> w872
          frame 0, Default {
          }
          frame 1 {
            n374 = Select(t=4.0, s=w1004, f=5.0) -> (s? t:f=w1005:dbl)
          }
          frame 2 {
            n375 = Select(t=4.0, s=w1011, f=5.0) -> (s? t:f=w1008:dbl)
          }
          frame 3 {
          }
        }
        n376 = case shown="0, Default" w890 {
          tunnel: w889 -> [_ w995 w1001 _]
          tunnel: [0.0 ("t") w994 w998 0.0 ("f")] -> w871
          frame 0, Default {
          }
          frame 1 {
            n377 = Select(t=4.0, s=w995, f=5.0) -> (s? t:f=w994:dbl)
          }
          frame 2 {
            n378 = Select(t=4.0, s=w1001, f=5.0) -> (s? t:f=w998:dbl)
          }
          frame 3 {
          }
        }
        n379 = case shown="0, Default" w888 {
          tunnel: w887 -> [_ w984 w991 _]
          tunnel: [0.0 ("t") w985 w988 0.0 ("f")] -> w870
          frame 0, Default {
          }
          frame 1 {
            n380 = Select(t=4.0, s=w984, f=5.0) -> (s? t:f=w985:dbl)
          }
          frame 2 {
            n381 = Select(t=4.0, s=w991, f=5.0) -> (s? t:f=w988:dbl)
          }
          frame 3 {
          }
        }
        n382 = case shown="0, Default" w886 {
          tunnel: w885 -> [_ w975 w981 _]
          tunnel: [0.0 ("t") w974 w978 0.0 ("f")] -> w869
          frame 0, Default {
          }
          frame 1 {
            n383 = Select(t=4.0, s=w975, f=5.0) -> (s? t:f=w974:dbl)
          }
          frame 2 {
            n384 = Select(t=4.0, s=w981, f=5.0) -> (s? t:f=w978:dbl)
          }
          frame 3 {
          }
        }
        n385 = case shown="0, Default" w884 {
          tunnel: w883 -> [_ w965 w971 _]
          tunnel: [0.0 ("t") w964 w968 0.0 ("f")] -> w868
          frame 0, Default {
          }
          frame 1 {
            n386 = Select(t=4.0, s=w965, f=5.0) -> (s? t:f=w964:dbl)
          }
          frame 2 {
            n387 = Select(t=4.0, s=w971, f=5.0) -> (s? t:f=w968:dbl)
          }
          frame 3 {
          }
        }
        n388 = case shown="0, Default" w882 {
          tunnel: w881 -> [_ w955 w961 _]
          tunnel: [0.0 ("t") w954 w958 0.0 ("f")] -> w867
          frame 0, Default {
          }
          frame 1 {
            n389 = Select(t=4.0, s=w955, f=5.0) -> (s? t:f=w954:dbl)
          }
          frame 2 {
            n390 = Select(t=4.0, s=w961, f=5.0) -> (s? t:f=w958:dbl)
          }
          frame 3 {
          }
        }
        n391 = case shown="0, Default" w880 {
          tunnel: w879 -> [_ w945 w951 _]
          tunnel: [0.0 ("t") w944 w948 0.0 ("f")] -> w866
          frame 0, Default {
          }
          frame 1 {
            n392 = Select(t=4.0, s=w945, f=5.0) -> (s? t:f=w944:dbl)
          }
          frame 2 {
            n393 = Select(t=4.0, s=w951, f=5.0) -> (s? t:f=w948:dbl)
          }
          frame 3 {
          }
        }
        n394 = case shown="0, Default" w878 {
          tunnel: w877 -> [_ w935 w941 _]
          tunnel: [0.0 ("t") w934 w938 0.0 ("f")] -> w865
          frame 0, Default {
          }
          frame 1 {
            n395 = Select(t=4.0, s=w935, f=5.0) -> (s? t:f=w934:dbl)
          }
          frame 2 {
            n396 = Select(t=4.0, s=w941, f=5.0) -> (s? t:f=w938:dbl)
          }
          frame 3 {
          }
        }
        n397 = case shown="0, Default" w876 {
          tunnel: w875 -> [_ w925 w931 _]
          tunnel: [0.0 ("t") w924 w928 0.0 ("f")] -> w864
          frame 0, Default {
          }
          frame 1 {
            n398 = Select(t=4.0, s=w925, f=5.0) -> (s? t:f=w924:dbl)
          }
          frame 2 {
            n399 = Select(t=4.0, s=w931, f=5.0) -> (s? t:f=w928:dbl)
          }
          frame 3 {
          }
        }
        n400 = case shown="0, Default" w874 {
          tunnel: w873 -> [_ w915 w921 _]
          tunnel: [0.0 ("t") w914 w918 0.0 ("f")] -> w855
          frame 0, Default {
          }
          frame 1 {
            n401 = Select(t=4.0, s=w915, f=5.0) -> (s? t:f=w914:dbl)
          }
          frame 2 {
            n402 = Select(t=4.0, s=w921, f=5.0) -> (s? t:f=w918:dbl)
          }
          frame 3 {
          }
        }
        n403 = call ".INI READ.vi"() -> ("MODE"=w850:string, "TEST MODE"=w853:string, "TIME"=w845:dbl)  [unwired: 4 in, 5 out]
        n404 = Equal?(x=w853, y="RETEST") -> (x = y?=w851:bool)
        n405 = case shown="False" w851 {
          tunnel: [1.0 ("element") 2.0 ("element")] -> w847
          frame False {
          }
          frame True {
          }
        }
        n406 = Equal?(x=w850, y="CHANNEL REF MODE") -> (x = y?=w848:bool)
        n407 = case shown="False" w848 {
          tunnel: [1.0 ("element") 2.0 ("element")] -> w846
          frame False {
          }
          frame True {
          }
        }
        n408 = Build Array(w844, w844, w844, w844, w844, w844, w847, w846, w844, w845, w844, w844, w844, w844, w844, w844, w844, w844, w844, w844, w844, w844, w844, w844, w844, w844, w844, w844, w844, w844, w844, w844, w844, w844, w844, w844, w844, w844, w844, w844, w872, w871, w870, w869, w868, w867, w866, w865, w864, w855, 0.0 ("element"), 187.0 ("element")) -> (w861:dbl[])
        n409 = flat-sequence {
          tunnel: w861 -> [w912]
          tunnel: [w912] -> w854
          frame #0 {
            n410 = Wait (ms)(milliseconds to wait=u32 0) -> ()  [unwired: 1 out]
          }
        }
        n411 = call-poly "VISA Configure Serial Port"("VISA resource name"=w863, "timeout (10sec)"=u32 2000, "baud rate (9600)"=u32 115200, "data bits (8)"=u16 8, "parity (0:none)"=enum16{"None", "Odd", "Even", "Mark", "Space"}."None", "stop bits (10: 1 bit)"=w859) -> ("VISA resource name out"=w904:refnum<visa-resource-name>, "error out"=w903:errorcluster)  [unwired: 8 in]
        n412 = VISA Open(timeout (0)=u32 2000 ("VISA Open timeout (0)"), error in (no error)=w903, VISA resource name=w904) -> (VISA resource name=w895:refnum<visa-resource-name>, error out=w896:errorcluster)  [unwired: 2 in]
        n413 = flat-sequence {
          tunnel: [w1015] -> w897
          tunnel: w896 -> [w1015]
          tunnel: w895 -> [w1014]
          tunnel: [w1014] -> w894
          frame #0 {
            n414 = Wait (ms)(milliseconds to wait=u32 0) -> ()  [unwired: 1 out]
          }
        }
        n415 = Byte Array To String(unsigned byte array=w854) -> (string=w856:string)
        n416 = VISA Write(VISA resource name=w894, write buffer=w856, error in (no error)=w897) -> (VISA resource name out=w899:refnum<visa-resource-name>, error out=w898:errorcluster)  [unwired: 1 out]
        n417 = VISA Close(VISA resource name=w899, error in (no error)=w898) -> (error out=w860:errorcluster)
      }
      frame "READY TO PRINT" {
        n418 = Unbundle By Name(w1024) -> ("RES VALUE 1"=w1021:dbl)
        n419 = call "Label Generation.vi"() -> ("error out 2"=w1019:errorcluster)  [unwired: 7 in, 4 out]
        n420 = Number To Decimal String(number=w1021) -> (decimal integer string=w1023:string)  [unwired: 1 in]
        n421 = case shown="No Error" w1019 {
          frame No Error {
            n422 = property on="Printer" class="Bool (strict)"("Colors [4]"=cluster{u32, u32}[] [{1244968, 65309}]) -> ()  [unwired: 2 in, 2 out]
          }
          frame Error {
            n423 = property on="Printer" class="Bool (strict)"("Colors [4]"=cluster{u32, u32}[] [{16720896, 16731178}]) -> ()  [unwired: 2 in, 2 out]
          }
        }
        n424 = call <userlib>:"String to 1D Array__ogtk.vi"("string"=w1023) -> ("Array of Strings"=w1022:string[])  [unwired: 10 in]
        n425 = call ".INI READ.vi"() -> ("Serail No"=w1017:cluster{"Serial Number":T5})  [unwired: 4 in, 7 out]
        n426 = Unbundle By Name(w1017) -> ("Serial Number"=w1016:T5)
        n427 = call "Update Serial Number1.vi"() -> ()  [unwired: 9 in, 3 out]
        n428 = call "Label Generation.vi"("Resistance Value"=w1022, "Serial No"=w1016) -> ("Printer Command"=→"Printer Command":string)  [unwired: 5 in, 4 out]
      }
      frame "REPORT " {
        n429 = call ".INI READ.vi"() -> ("MODE"=w1027:string, "TEST MODE"=w1028:string)  [unwired: 4 in, 6 out]
        n430 = Equal?(x=w1028, y="RETEST") -> (x = y?=w1030:bool)
        n431 = call "Report Gen Title_Folder.vi"() -> ("appended path"=w1034:path)  [unwired: 11 in]
        n432 = Select(t=TRUE, s=w1030, f=FALSE) -> (s? t:f=w1029:bool)
        n433 = stacked-sequence {
          tunnel: w1035 -> [w1041 w1120 w1199 w1278 w1357 w1436 w1515 w1594 w1673 w1752]
          tunnel: w1034 -> [w1040 w1119 w1198 w1277 w1356 w1435 w1514 w1593 w1672 w1751]
          tunnel: w1029 -> [w1039 w1118 w1197 w1276 w1355 w1434 w1513 w1592 w1671 w1750]
          tunnel: w1029 -> [w1038 w1116 w1195 w1274 w1353 w1432 w1511 w1590 w1669 w1748]
          tunnel: w1027 -> [w1037 w1117 w1196 w1275 w1354 w1433 w1512 w1591 w1670 w1749]
          frame #0 {
            # "Channel 1 data log"
            n434 = Unbundle By Name(w1041) -> ("PP 1"=w1042:i32)
            n435 = case shown="1" w1042 {
              tunnel: w1041 -> [_ w1052 w1078]
              tunnel: w1040 -> [_ w1053 w1081]
              tunnel: w1039 -> [_ w1045 w1080]
              tunnel: w1038 -> [_ _ w1079]
              tunnel: w1037 -> [_ w1044 w1077]
              frame 0, Default {
              }
              frame 1 {
                n436 = Unbundle By Name(w1052) -> ("SET VALUE 1"=w1072:dbl, "TOL 1"=w1070:dbl, "RES VALUE 1"=w1068:dbl, "CH  PASS  1"=w1066:bool, "CH1 MAX TOL"=w1051:dbl, "CH1 MIN TOL"=w1049:dbl)
                n437 = case shown="True" w1066 {
                  tunnel: ["FAIL" "PASS"] -> w1059
                  frame False {
                  }
                  frame True {
                  }
                }
                n438 = case shown="True" w1045 {
                  tunnel: ["NORMAL" "RETEST"] -> w1043
                  frame False {
                  }
                  frame True {
                  }
                }
                n439 = Get Date/Time String() -> (date string=w1064:string, time string=w1065:string)  [unwired: 3 in]
                n440 = Concatenate Strings(w1064, w1065) -> (w1063:string)
                n441 = Number To Fractional String(number=w1051, precision (6)=i16 3) -> (F-format string=w1047:string)  [unwired: 2 in]
                n442 = Number To Fractional String(number=w1072, precision (6)=i16 3 ("width (-)")) -> (F-format string=w1062:string)  [unwired: 2 in]
                n443 = Number To Fractional String(number=w1070, precision (6)=i16 3 ("width (-)")) -> (F-format string=w1061:string)  [unwired: 2 in]
                n444 = Number To Fractional String(number=w1068, precision (6)=i16 3 ("width (-)")) -> (F-format string=w1060:string)  [unwired: 2 in]
                n445 = Number To Fractional String(number=w1049, precision (6)=i16 3) -> (F-format string=w1046:string)  [unwired: 2 in]
                n446 = Build Array(w1063, w1062, w1061, w1060, w1059, "1" ("element"), w1047, w1046, w1044, w1043) -> (w1057:string[])
                n447 = call-poly <vilib>:"Write Delimited Spreadsheet.vi"("file path (dialog if empty)"=w1053, "1D data"=w1057, "append to file? (new file:F)"=TRUE, "transpose? (no:F)"=FALSE, "delimiter (\\t)"="," ("delimiter (\\t)")) -> ()  [unwired: 9 in, 2 out]
              }
              frame 2 {
                n448 = case shown="True" w1079 {
                  tunnel: w1081 -> [_ w1086]
                  tunnel: w1080 -> [_ w1085]
                  tunnel: w1078 -> [_ w1084]
                  tunnel: w1077 -> [_ w1083]
                  frame False {
                  }
                  frame True {
                    n449 = Unbundle By Name(w1084) -> ("SET VALUE 1"=w1111:dbl, "TOL 1"=w1109:dbl, "RES VALUE 1"=w1107:dbl, "CH  PASS  1"=w1105:bool, "CH1 MAX TOL"=w1092:dbl, "CH1 MIN TOL"=w1090:dbl)
                    n450 = case shown="False" w1105 {
                      tunnel: ["FAIL" "PASS"] -> w1098
                      frame False {
                      }
                      frame True {
                      }
                    }
                    n451 = case shown="True" w1085 {
                      tunnel: ["NORMAL" "RETEST"] -> w1082
                      frame False {
                      }
                      frame True {
                      }
                    }
                    n452 = Get Date/Time String() -> (date string=w1103:string, time string=w1104:string)  [unwired: 3 in]
                    n453 = Concatenate Strings(w1103, w1104) -> (w1102:string)
                    n454 = Number To Fractional String(number=w1092, precision (6)=i16 3) -> (F-format string=w1088:string)  [unwired: 2 in]
                    n455 = Number To Fractional String(number=w1111, precision (6)=i16 3 ("width (-)")) -> (F-format string=w1101:string)  [unwired: 2 in]
                    n456 = Number To Fractional String(number=w1109, precision (6)=i16 3 ("width (-)")) -> (F-format string=w1100:string)  [unwired: 2 in]
                    n457 = Number To Fractional String(number=w1107, precision (6)=i16 3 ("width (-)")) -> (F-format string=w1099:string)  [unwired: 2 in]
                    n458 = Number To Fractional String(number=w1090, precision (6)=i16 3) -> (F-format string=w1087:string)  [unwired: 2 in]
                    n459 = Build Array(w1102, w1101, w1100, w1099, w1098, "1" ("element"), w1088, w1087, w1083, w1082) -> (w1096:string[])
                    n460 = call-poly <vilib>:"Write Delimited Spreadsheet.vi"("file path (dialog if empty)"=w1086, "1D data"=w1096, "append to file? (new file:F)"=TRUE, "transpose? (no:F)"=FALSE, "delimiter (\\t)"="," ("delimiter (\\t)")) -> ()  [unwired: 9 in, 2 out]
                  }
                }
              }
            }
          }
          frame #1 {
            # "CHANNEL 2 DATA LOG"
            n461 = Unbundle By Name(w1120) -> ("PP 2"=w1121:i32)
            n462 = case shown="1" w1121 {
              tunnel: w1120 -> [_ w1143 w1156]
              tunnel: w1119 -> [_ w1134 w1157]
              tunnel: w1118 -> [_ w1124 w1159]
              tunnel: w1117 -> [_ w1123 w1160]
              tunnel: w1116 -> [_ _ w1158]
              frame 0, Default {
              }
              frame 1 {
                n463 = Unbundle By Name(w1143) -> ("SET VALUE 2"=w1151:dbl, "TOL 2"=w1149:dbl, "RES VALUE 2"=w1147:dbl, "CH  PASS 2"=w1145:bool, "CH2 MAX TOL"=w1130:dbl, "CH2 MIN TOL"=w1129:dbl)
                n464 = case shown="False" w1145 {
                  tunnel: ["FAIL" "PASS"] -> w1137
                  frame False {
                  }
                  frame True {
                  }
                }
                n465 = case shown="True" w1124 {
                  tunnel: ["NORMAL" "RETEST"] -> w1122
                  frame False {
                  }
                  frame True {
                  }
                }
                n466 = Get Date/Time String() -> (date string=w1142:string, time string=w1144:string)  [unwired: 3 in]
                n467 = Concatenate Strings(w1142, w1144) -> (w1141:string)
                n468 = Number To Fractional String(number=w1130, precision (6)=i16 3) -> (F-format string=w1126:string)  [unwired: 2 in]
                n469 = Number To Fractional String(number=w1151, precision (6)=i16 3 ("width (-)")) -> (F-format string=w1140:string)  [unwired: 2 in]
                n470 = Number To Fractional String(number=w1149, precision (6)=i16 3 ("width (-)")) -> (F-format string=w1139:string)  [unwired: 2 in]
                n471 = Number To Fractional String(number=w1147, precision (6)=i16 3 ("width (-)")) -> (F-format string=w1138:string)  [unwired: 2 in]
                n472 = Number To Fractional String(number=w1129, precision (6)=i16 3) -> (F-format string=w1125:string)  [unwired: 2 in]
                n473 = Build Array(w1141, w1140, w1139, w1138, w1137, "2" ("element"), w1126, w1125, w1123, w1122) -> (w1135:string[])
                n474 = call-poly <vilib>:"Write Delimited Spreadsheet.vi"("file path (dialog if empty)"=w1134, "1D data"=w1135, "append to file? (new file:F)"=TRUE, "transpose? (no:F)"=FALSE, "delimiter (\\t)"="," ("delimiter (\\t)")) -> ()  [unwired: 9 in, 2 out]
              }
              frame 2 {
                n475 = case shown="False" w1158 {
                  tunnel: w1160 -> [_ w1164]
                  tunnel: w1159 -> [_ w1163]
                  tunnel: w1157 -> [_ w1162]
                  tunnel: w1156 -> [_ w1161]
                  frame False {
                  }
                  frame True {
                    n476 = Unbundle By Name(w1161) -> ("SET VALUE 2"=w1190:dbl, "TOL 2"=w1188:dbl, "RES VALUE 2"=w1186:dbl, "CH  PASS 2"=w1184:bool, "CH2 MAX TOL"=w1171:dbl, "CH2 MIN TOL"=w1170:dbl)
                    n477 = case shown="False" w1184 {
                      tunnel: ["FAIL" "PASS"] -> w1177
                      frame False {
                      }
                      frame True {
                      }
                    }
                    n478 = case shown="True" w1163 {
                      tunnel: ["NORMAL" "RETEST"] -> w1165
                      frame False {
                      }
                      frame True {
                      }
                    }
                    n479 = Get Date/Time String() -> (date string=w1182:string, time string=w1183:string)  [unwired: 3 in]
                    n480 = Concatenate Strings(w1182, w1183) -> (w1181:string)
                    n481 = Number To Fractional String(number=w1171, precision (6)=i16 3) -> (F-format string=w1167:string)  [unwired: 2 in]
                    n482 = Number To Fractional String(number=w1190, precision (6)=i16 3 ("width (-)")) -> (F-format string=w1180:string)  [unwired: 2 in]
                    n483 = Number To Fractional String(number=w1188, precision (6)=i16 3 ("width (-)")) -> (F-format string=w1179:string)  [unwired: 2 in]
                    n484 = Number To Fractional String(number=w1186, precision (6)=i16 3 ("width (-)")) -> (F-format string=w1178:string)  [unwired: 2 in]
                    n485 = Number To Fractional String(number=w1170, precision (6)=i16 3) -> (F-format string=w1166:string)  [unwired: 2 in]
                    n486 = Build Array(w1181, w1180, w1179, w1178, w1177, "2" ("element"), w1167, w1166, w1164, w1165) -> (w1175:string[])
                    n487 = call-poly <vilib>:"Write Delimited Spreadsheet.vi"("file path (dialog if empty)"=w1162, "1D data"=w1175, "append to file? (new file:F)"=TRUE, "transpose? (no:F)"=FALSE, "delimiter (\\t)"="," ("delimiter (\\t)")) -> ()  [unwired: 9 in, 2 out]
                  }
                }
              }
            }
          }
          frame #2 {
            # "Channel 3 data log"
            n488 = Unbundle By Name(w1199) -> ("PP 3"=w1200:i32)
            n489 = case shown="0, Default" w1200 {
              tunnel: w1199 -> [_ w1210 w1235]
              tunnel: w1198 -> [_ w1211 w1239]
              tunnel: w1197 -> [_ w1203 w1237]
              tunnel: w1196 -> [_ w1202 w1238]
              tunnel: w1195 -> [_ _ w1236]
              frame 0, Default {
              }
              frame 1 {
                n490 = Unbundle By Name(w1210) -> ("SET VALUE 3"=w1230:dbl, "TOL 3"=w1228:dbl, "RES VALUE 3"=w1226:dbl, "CH  PASS 3"=w1224:bool, "CH3 MAX TOL"=w1209:dbl, "CH3 MIN TOL"=w1208:dbl)
                n491 = case shown="False" w1224 {
                  tunnel: ["FAIL" "PASS"] -> w1217
                  frame False {
                  }
                  frame True {
                  }
                }
                n492 = case shown="True" w1203 {
                  tunnel: ["NORMAL" "RETEST"] -> w1201
                  frame False {
                  }
                  frame True {
                  }
                }
                n493 = Get Date/Time String() -> (date string=w1222:string, time string=w1223:string)  [unwired: 3 in]
                n494 = Concatenate Strings(w1222, w1223) -> (w1221:string)
                n495 = Number To Fractional String(number=w1230, precision (6)=i16 3 ("width (-)")) -> (F-format string=w1220:string)  [unwired: 2 in]
                n496 = Number To Fractional String(number=w1228, precision (6)=i16 3 ("width (-)")) -> (F-format string=w1219:string)  [unwired: 2 in]
                n497 = Number To Fractional String(number=w1226, precision (6)=i16 3 ("width (-)")) -> (F-format string=w1218:string)  [unwired: 2 in]
                n498 = Number To Fractional String(number=w1209, precision (6)=i16 3) -> (F-format string=w1205:string)  [unwired: 2 in]
                n499 = Number To Fractional String(number=w1208, precision (6)=i16 3) -> (F-format string=w1204:string)  [unwired: 2 in]
                n500 = Build Array(w1221, w1220, w1219, w1218, w1217, "3" ("element"), w1205, w1204, w1202, w1201) -> (w1215:string[])
                n501 = call-poly <vilib>:"Write Delimited Spreadsheet.vi"("file path (dialog if empty)"=w1211, "1D data"=w1215, "append to file? (new file:F)"=TRUE, "transpose? (no:F)"=FALSE, "delimiter (\\t)"="," ("delimiter (\\t)")) -> ()  [unwired: 9 in, 2 out]
              }
              frame 2 {
                n502 = case shown="True" w1236 {
                  tunnel: w1239 -> [_ w1243]
                  tunnel: w1238 -> [_ w1242]
                  tunnel: w1237 -> [_ w1241]
                  tunnel: w1235 -> [_ w1240]
                  frame False {
                  }
                  frame True {
                    n503 = Unbundle By Name(w1240) -> ("SET VALUE 3"=w1269:dbl, "TOL 3"=w1267:dbl, "RES VALUE 3"=w1265:dbl, "CH  PASS 3"=w1263:bool, "CH3 MAX TOL"=w1250:dbl, "CH3 MIN TOL"=w1249:dbl)
                    n504 = case shown="False" w1263 {
                      tunnel: ["FAIL" "PASS"] -> w1256
                      frame False {
                      }
                      frame True {
                      }
                    }
                    n505 = case shown="True" w1241 {
                      tunnel: ["NORMAL" "RETEST"] -> w1244
                      frame False {
                      }
                      frame True {
                      }
                    }
                    n506 = Get Date/Time String() -> (date string=w1261:string, time string=w1262:string)  [unwired: 3 in]
                    n507 = Concatenate Strings(w1261, w1262) -> (w1260:string)
                    n508 = Number To Fractional String(number=w1269, precision (6)=i16 3 ("width (-)")) -> (F-format string=w1259:string)  [unwired: 2 in]
                    n509 = Number To Fractional String(number=w1267, precision (6)=i16 3 ("width (-)")) -> (F-format string=w1258:string)  [unwired: 2 in]
                    n510 = Number To Fractional String(number=w1265, precision (6)=i16 3 ("width (-)")) -> (F-format string=w1257:string)  [unwired: 2 in]
                    n511 = Number To Fractional String(number=w1250, precision (6)=i16 3) -> (F-format string=w1246:string)  [unwired: 2 in]
                    n512 = Number To Fractional String(number=w1249, precision (6)=i16 3) -> (F-format string=w1245:string)  [unwired: 2 in]
                    n513 = Build Array(w1260, w1259, w1258, w1257, w1256, "3" ("element"), w1246, w1245, w1242, w1244) -> (w1254:string[])
                    n514 = call-poly <vilib>:"Write Delimited Spreadsheet.vi"("file path (dialog if empty)"=w1243, "1D data"=w1254, "append to file? (new file:F)"=TRUE, "transpose? (no:F)"=FALSE, "delimiter (\\t)"="," ("delimiter (\\t)")) -> ()  [unwired: 9 in, 2 out]
                  }
                }
              }
            }
          }
          frame #3 {
            # "Channel 4 data log"
            n515 = Unbundle By Name(w1278) -> ("PP 4"=w1279:i32)
            n516 = case shown="0, Default" w1279 {
              tunnel: w1278 -> [_ w1289 w1315]
              tunnel: w1277 -> [_ w1290 w1316]
              tunnel: w1276 -> [_ w1282 w1317]
              tunnel: w1275 -> [_ w1281 w1318]
              tunnel: w1274 -> [_ _ w1314]
              frame 0, Default {
              }
              frame 1 {
                n517 = Unbundle By Name(w1289) -> ("SET VALUE 4"=w1309:dbl, "TOL 4"=w1307:dbl, "RES VALUE 4"=w1305:dbl, "CH  PASS 4"=w1303:bool, "CH4 MAX TOL"=w1288:dbl, "CH4 MIN TOL"=w1285:dbl)
                n518 = case shown="False" w1303 {
                  tunnel: ["FAIL" "PASS"] -> w1296
                  frame False {
                  }
                  frame True {
                  }
                }
                n519 = case shown="True" w1282 {
                  tunnel: ["NORMAL" "RETEST"] -> w1280
                  frame False {
                  }
                  frame True {
                  }
                }
                n520 = Get Date/Time String() -> (date string=w1301:string, time string=w1302:string)  [unwired: 3 in]
                n521 = Concatenate Strings(w1301, w1302) -> (w1300:string)
                n522 = Number To Fractional String(number=w1285, precision (6)=i16 3) -> (F-format string=w1283:string)  [unwired: 2 in]
                n523 = Number To Fractional String(number=w1309, precision (6)=i16 3 ("width (-)")) -> (F-format string=w1299:string)  [unwired: 2 in]
                n524 = Number To Fractional String(number=w1307, precision (6)=i16 3 ("width (-)")) -> (F-format string=w1298:string)  [unwired: 2 in]
                n525 = Number To Fractional String(number=w1305, precision (6)=i16 3 ("width (-)")) -> (F-format string=w1297:string)  [unwired: 2 in]
                n526 = Number To Fractional String(number=w1288, precision (6)=i16 3) -> (F-format string=w1286:string)  [unwired: 2 in]
                n527 = Build Array(w1300, w1299, w1298, w1297, w1296, "4" ("element"), w1286, w1283, w1281, w1280) -> (w1294:string[])
                n528 = call-poly <vilib>:"Write Delimited Spreadsheet.vi"("file path (dialog if empty)"=w1290, "1D data"=w1294, "append to file? (new file:F)"=TRUE, "transpose? (no:F)"=FALSE, "delimiter (\\t)"="," ("delimiter (\\t)")) -> ()  [unwired: 9 in, 2 out]
              }
              frame 2 {
                n529 = case shown="False" w1314 {
                  tunnel: w1318 -> [_ w1322]
                  tunnel: w1317 -> [_ w1321]
                  tunnel: w1316 -> [_ w1320]
                  tunnel: w1315 -> [_ w1319]
                  frame False {
                  }
                  frame True {
                    n530 = Unbundle By Name(w1319) -> ("SET VALUE 4"=w1348:dbl, "TOL 4"=w1346:dbl, "RES VALUE 4"=w1344:dbl, "CH  PASS 4"=w1342:bool, "CH4 MAX TOL"=w1329:dbl, "CH4 MIN TOL"=w1326:dbl)
                    n531 = case shown="False" w1342 {
                      tunnel: ["FAIL" "PASS"] -> w1335
                      frame False {
                      }
                      frame True {
                      }
                    }
                    n532 = case shown="True" w1321 {
                      tunnel: ["NORMAL" "RETEST"] -> w1323
                      frame False {
                      }
                      frame True {
                      }
                    }
                    n533 = Get Date/Time String() -> (date string=w1340:string, time string=w1341:string)  [unwired: 3 in]
                    n534 = Concatenate Strings(w1340, w1341) -> (w1339:string)
                    n535 = Number To Fractional String(number=w1326, precision (6)=i16 3) -> (F-format string=w1324:string)  [unwired: 2 in]
                    n536 = Number To Fractional String(number=w1348, precision (6)=i16 3 ("width (-)")) -> (F-format string=w1338:string)  [unwired: 2 in]
                    n537 = Number To Fractional String(number=w1346, precision (6)=i16 3 ("width (-)")) -> (F-format string=w1337:string)  [unwired: 2 in]
                    n538 = Number To Fractional String(number=w1344, precision (6)=i16 3 ("width (-)")) -> (F-format string=w1336:string)  [unwired: 2 in]
                    n539 = Number To Fractional String(number=w1329, precision (6)=i16 3) -> (F-format string=w1327:string)  [unwired: 2 in]
                    n540 = Build Array(w1339, w1338, w1337, w1336, w1335, "4" ("element"), w1327, w1324, w1322, w1323) -> (w1333:string[])
                    n541 = call-poly <vilib>:"Write Delimited Spreadsheet.vi"("file path (dialog if empty)"=w1320, "1D data"=w1333, "append to file? (new file:F)"=TRUE, "transpose? (no:F)"=FALSE, "delimiter (\\t)"="," ("delimiter (\\t)")) -> ()  [unwired: 9 in, 2 out]
                  }
                }
              }
            }
          }
          frame #4 {
            # "Channel 5 data log"
            n542 = Unbundle By Name(w1357) -> ("PP 5"=w1358:i32)
            n543 = case shown="2" w1358 {
              tunnel: w1357 -> [_ w1368 w1394]
              tunnel: w1356 -> [_ w1369 w1395]
              tunnel: w1355 -> [_ w1363 w1396]
              tunnel: w1354 -> [_ w1360 w1397]
              tunnel: w1353 -> [_ _ w1393]
              frame 0, Default {
              }
              frame 1 {
                n544 = Unbundle By Name(w1368) -> ("SET VALUE 5"=w1388:dbl, "TOL 5"=w1386:dbl, "RES VALUE 5"=w1384:dbl, "CH  PASS 5"=w1382:bool, "CH5 MAX TOL"=w1367:dbl, "CH5 MIN TOL"=w1365:dbl)
                n545 = case shown="False" w1382 {
                  tunnel: ["FAIL" "PASS"] -> w1375
                  frame False {
                  }
                  frame True {
                  }
                }
                n546 = case shown="True" w1363 {
                  tunnel: ["NORMAL" "RETEST"] -> w1359
                  frame False {
                  }
                  frame True {
                  }
                }
                n547 = Get Date/Time String() -> (date string=w1380:string, time string=w1381:string)  [unwired: 3 in]
                n548 = Concatenate Strings(w1380, w1381) -> (w1379:string)
                n549 = Number To Fractional String(number=w1388, precision (6)=i16 3 ("width (-)")) -> (F-format string=w1378:string)  [unwired: 2 in]
                n550 = Number To Fractional String(number=w1386, precision (6)=i16 3 ("width (-)")) -> (F-format string=w1377:string)  [unwired: 2 in]
                n551 = Number To Fractional String(number=w1384, precision (6)=i16 3 ("width (-)")) -> (F-format string=w1376:string)  [unwired: 2 in]
                n552 = Number To Fractional String(number=w1367, precision (6)=i16 3) -> (F-format string=w1362:string)  [unwired: 2 in]
                n553 = Number To Fractional String(number=w1365, precision (6)=i16 3) -> (F-format string=w1361:string)  [unwired: 2 in]
                n554 = Build Array(w1379, w1378, w1377, w1376, w1375, "5" ("element"), w1362, w1361, w1360, w1359) -> (w1373:string[])
                n555 = call-poly <vilib>:"Write Delimited Spreadsheet.vi"("file path (dialog if empty)"=w1369, "1D data"=w1373, "append to file? (new file:F)"=TRUE, "transpose? (no:F)"=FALSE, "delimiter (\\t)"="," ("delimiter (\\t)")) -> ()  [unwired: 9 in, 2 out]
              }
              frame 2 {
                n556 = case shown="True" w1393 {
                  tunnel: w1397 -> [_ w1401]
                  tunnel: w1396 -> [_ w1400]
                  tunnel: w1395 -> [_ w1399]
                  tunnel: w1394 -> [_ w1398]
                  frame False {
                  }
                  frame True {
                    n557 = Unbundle By Name(w1398) -> ("SET VALUE 5"=w1427:dbl, "TOL 5"=w1425:dbl, "RES VALUE 5"=w1423:dbl, "CH  PASS 5"=w1421:bool, "CH5 MAX TOL"=w1408:dbl, "CH5 MIN TOL"=w1406:dbl)
                    n558 = case shown="False" w1421 {
                      tunnel: ["FAIL" "PASS"] -> w1414
                      frame False {
                      }
                      frame True {
                      }
                    }
                    n559 = case shown="True" w1400 {
                      tunnel: ["NORMAL" "RETEST"] -> w1402
                      frame False {
                      }
                      frame True {
                      }
                    }
                    n560 = Get Date/Time String() -> (date string=w1419:string, time string=w1420:string)  [unwired: 3 in]
                    n561 = Concatenate Strings(w1419, w1420) -> (w1418:string)
                    n562 = Number To Fractional String(number=w1427, precision (6)=i16 3 ("width (-)")) -> (F-format string=w1417:string)  [unwired: 2 in]
                    n563 = Number To Fractional String(number=w1425, precision (6)=i16 3 ("width (-)")) -> (F-format string=w1416:string)  [unwired: 2 in]
                    n564 = Number To Fractional String(number=w1423, precision (6)=i16 3 ("width (-)")) -> (F-format string=w1415:string)  [unwired: 2 in]
                    n565 = Number To Fractional String(number=w1408, precision (6)=i16 3) -> (F-format string=w1404:string)  [unwired: 2 in]
                    n566 = Number To Fractional String(number=w1406, precision (6)=i16 3) -> (F-format string=w1403:string)  [unwired: 2 in]
                    n567 = Build Array(w1418, w1417, w1416, w1415, w1414, "5" ("element"), w1404, w1403, w1401, w1402) -> (w1412:string[])
                    n568 = call-poly <vilib>:"Write Delimited Spreadsheet.vi"("file path (dialog if empty)"=w1399, "1D data"=w1412, "append to file? (new file:F)"=TRUE, "transpose? (no:F)"=FALSE, "delimiter (\\t)"="," ("delimiter (\\t)")) -> ()  [unwired: 9 in, 2 out]
                  }
                }
              }
            }
          }
          frame #5 {
            # "Channel 6 data log"
            n569 = Unbundle By Name(w1436) -> ("PP 6"=w1437:i32)
            n570 = case shown="2" w1437 {
              tunnel: w1436 -> [_ w1447 w1473]
              tunnel: w1435 -> [_ w1448 w1474]
              tunnel: w1434 -> [_ w1440 w1476]
              tunnel: w1433 -> [_ w1439 w1475]
              tunnel: w1432 -> [_ _ w1472]
              frame 0, Default {
              }
              frame 1 {
                n571 = Unbundle By Name(w1447) -> ("SET VALUE 6"=w1467:dbl, "TOL 6"=w1465:dbl, "RES VALUE 6"=w1463:dbl, "CH  PASS 6"=w1461:bool, "CH6 MAX TOL"=w1444:dbl, "CH6 MIN TOL"=w1443:dbl)
                n572 = case shown="False" w1461 {
                  tunnel: ["FAIL" "PASS"] -> w1454
                  frame False {
                  }
                  frame True {
                  }
                }
                n573 = case shown="True" w1440 {
                  tunnel: ["NORMAL" "RETEST"] -> w1438
                  frame False {
                  }
                  frame True {
                  }
                }
                n574 = Get Date/Time String() -> (date string=w1459:string, time string=w1460:string)  [unwired: 3 in]
                n575 = Concatenate Strings(w1459, w1460) -> (w1458:string)
                n576 = Number To Fractional String(number=w1467, precision (6)=i16 3 ("width (-)")) -> (F-format string=w1457:string)  [unwired: 2 in]
                n577 = Number To Fractional String(number=w1465, precision (6)=i16 3 ("width (-)")) -> (F-format string=w1456:string)  [unwired: 2 in]
                n578 = Number To Fractional String(number=w1463, precision (6)=i16 3 ("width (-)")) -> (F-format string=w1455:string)  [unwired: 2 in]
                n579 = Number To Fractional String(number=w1444, precision (6)=i16 3) -> (F-format string=w1442:string)  [unwired: 2 in]
                n580 = Number To Fractional String(number=w1443, precision (6)=i16 3) -> (F-format string=w1441:string)  [unwired: 2 in]
                n581 = Build Array(w1458, w1457, w1456, w1455, w1454, "6" ("element"), w1442, w1441, w1439, w1438) -> (w1452:string[])
                n582 = call-poly <vilib>:"Write Delimited Spreadsheet.vi"("file path (dialog if empty)"=w1448, "1D data"=w1452, "append to file? (new file:F)"=TRUE, "transpose? (no:F)"=FALSE, "delimiter (\\t)"="," ("delimiter (\\t)")) -> ()  [unwired: 9 in, 2 out]
              }
              frame 2 {
                n583 = case shown="True" w1472 {
                  tunnel: w1476 -> [_ w1480]
                  tunnel: w1475 -> [_ w1479]
                  tunnel: w1474 -> [_ w1478]
                  tunnel: w1473 -> [_ w1477]
                  frame False {
                  }
                  frame True {
                    n584 = Unbundle By Name(w1477) -> ("SET VALUE 6"=w1506:dbl, "TOL 6"=w1504:dbl, "RES VALUE 6"=w1502:dbl, "CH  PASS 6"=w1500:bool, "CH6 MAX TOL"=w1485:dbl, "CH6 MIN TOL"=w1484:dbl)
                    n585 = case shown="False" w1500 {
                      tunnel: ["FAIL" "PASS"] -> w1493
                      frame False {
                      }
                      frame True {
                      }
                    }
                    n586 = case shown="True" w1480 {
                      tunnel: ["NORMAL" "RETEST"] -> w1481
                      frame False {
                      }
                      frame True {
                      }
                    }
                    n587 = Get Date/Time String() -> (date string=w1498:string, time string=w1499:string)  [unwired: 3 in]
                    n588 = Concatenate Strings(w1498, w1499) -> (w1497:string)
                    n589 = Number To Fractional String(number=w1506, precision (6)=i16 3 ("width (-)")) -> (F-format string=w1496:string)  [unwired: 2 in]
                    n590 = Number To Fractional String(number=w1504, precision (6)=i16 3 ("width (-)")) -> (F-format string=w1495:string)  [unwired: 2 in]
                    n591 = Number To Fractional String(number=w1502, precision (6)=i16 3 ("width (-)")) -> (F-format string=w1494:string)  [unwired: 2 in]
                    n592 = Number To Fractional String(number=w1485, precision (6)=i16 3) -> (F-format string=w1483:string)  [unwired: 2 in]
                    n593 = Number To Fractional String(number=w1484, precision (6)=i16 3) -> (F-format string=w1482:string)  [unwired: 2 in]
                    n594 = Build Array(w1497, w1496, w1495, w1494, w1493, "6" ("element"), w1483, w1482, w1479, w1481) -> (w1491:string[])
                    n595 = call-poly <vilib>:"Write Delimited Spreadsheet.vi"("file path (dialog if empty)"=w1478, "1D data"=w1491, "append to file? (new file:F)"=TRUE, "transpose? (no:F)"=FALSE, "delimiter (\\t)"="," ("delimiter (\\t)")) -> ()  [unwired: 9 in, 2 out]
                  }
                }
              }
            }
          }
          frame #6 {
            # "Channel 7 data log"
            n596 = Unbundle By Name(w1515) -> ("PP 7"=w1516:i32)
            n597 = case shown="2" w1516 {
              tunnel: w1515 -> [_ w1526 w1551]
              tunnel: w1514 -> [_ w1527 w1554]
              tunnel: w1513 -> [_ w1519 w1552]
              tunnel: w1512 -> [_ w1518 w1553]
              tunnel: w1511 -> [_ _ w1555]
              frame 0, Default {
              }
              frame 1 {
                n598 = Unbundle By Name(w1526) -> ("SET VALUE 7"=w1546:dbl, "TOL 7"=w1544:dbl, "RES VALUE 7"=w1542:dbl, "CH  PASS 7"=w1540:bool, "CH7 MAX TOL"=w1525:dbl, "CH7 MIN TOL"=w1523:dbl)
                n599 = case shown="False" w1540 {
                  tunnel: ["FAIL" "PASS"] -> w1533
                  frame False {
                  }
                  frame True {
                  }
                }
                n600 = case shown="False" w1519 {
                  tunnel: ["NORMAL" "RETEST"] -> w1517
                  frame False {
                  }
                  frame True {
                  }
                }
                n601 = Get Date/Time String() -> (date string=w1538:string, time string=w1539:string)  [unwired: 3 in]
                n602 = Concatenate Strings(w1538, w1539) -> (w1537:string)
                n603 = Number To Fractional String(number=w1546, precision (6)=i16 3 ("width (-)")) -> (F-format string=w1536:string)  [unwired: 2 in]
                n604 = Number To Fractional String(number=w1544, precision (6)=i16 3 ("width (-)")) -> (F-format string=w1535:string)  [unwired: 2 in]
                n605 = Number To Fractional String(number=w1542, precision (6)=i16 3 ("width (-)")) -> (F-format string=w1534:string)  [unwired: 2 in]
                n606 = Number To Fractional String(number=w1525, precision (6)=i16 3) -> (F-format string=w1521:string)  [unwired: 2 in]
                n607 = Number To Fractional String(number=w1523, precision (6)=i16 3) -> (F-format string=w1520:string)  [unwired: 2 in]
                n608 = Build Array(w1537, w1536, w1535, w1534, w1533, "7" ("element"), w1521, w1520, w1518, w1517) -> (w1531:string[])
                n609 = call-poly <vilib>:"Write Delimited Spreadsheet.vi"("file path (dialog if empty)"=w1527, "1D data"=w1531, "append to file? (new file:F)"=TRUE, "transpose? (no:F)"=FALSE, "delimiter (\\t)"="," ("delimiter (\\t)")) -> ()  [unwired: 9 in, 2 out]
              }
              frame 2 {
                n610 = case shown="True" w1555 {
                  tunnel: w1554 -> [_ w1559]
                  tunnel: w1553 -> [_ w1558]
                  tunnel: w1552 -> [_ w1557]
                  tunnel: w1551 -> [_ w1556]
                  frame False {
                  }
                  frame True {
                    n611 = Unbundle By Name(w1556) -> ("SET VALUE 7"=w1585:dbl, "TOL 7"=w1583:dbl, "RES VALUE 7"=w1581:dbl, "CH  PASS 7"=w1579:bool, "CH7 MAX TOL"=w1566:dbl, "CH7 MIN TOL"=w1564:dbl)
                    n612 = case shown="False" w1579 {
                      tunnel: ["FAIL" "PASS"] -> w1572
                      frame False {
                      }
                      frame True {
                      }
                    }
                    n613 = case shown="False" w1557 {
                      tunnel: ["NORMAL" "RETEST"] -> w1560
                      frame False {
                      }
                      frame True {
                      }
                    }
                    n614 = Get Date/Time String() -> (date string=w1577:string, time string=w1578:string)  [unwired: 3 in]
                    n615 = Concatenate Strings(w1577, w1578) -> (w1576:string)
                    n616 = Number To Fractional String(number=w1585, precision (6)=i16 3 ("width (-)")) -> (F-format string=w1575:string)  [unwired: 2 in]
                    n617 = Number To Fractional String(number=w1583, precision (6)=i16 3 ("width (-)")) -> (F-format string=w1574:string)  [unwired: 2 in]
                    n618 = Number To Fractional String(number=w1581, precision (6)=i16 3 ("width (-)")) -> (F-format string=w1573:string)  [unwired: 2 in]
                    n619 = Number To Fractional String(number=w1566, precision (6)=i16 3) -> (F-format string=w1562:string)  [unwired: 2 in]
                    n620 = Number To Fractional String(number=w1564, precision (6)=i16 3) -> (F-format string=w1561:string)  [unwired: 2 in]
                    n621 = Build Array(w1576, w1575, w1574, w1573, w1572, "7" ("element"), w1562, w1561, w1558, w1560) -> (w1570:string[])
                    n622 = call-poly <vilib>:"Write Delimited Spreadsheet.vi"("file path (dialog if empty)"=w1559, "1D data"=w1570, "append to file? (new file:F)"=TRUE, "transpose? (no:F)"=FALSE, "delimiter (\\t)"="," ("delimiter (\\t)")) -> ()  [unwired: 9 in, 2 out]
                  }
                }
              }
            }
          }
          frame #7 {
            # "Channel 8 data log"
            n623 = Unbundle By Name(w1594) -> ("PP 8"=w1595:i32)
            n624 = case shown="2" w1595 {
              tunnel: w1594 -> [_ w1605 w1633]
              tunnel: w1593 -> [_ w1606 w1634]
              tunnel: w1592 -> [_ w1600 w1631]
              tunnel: w1591 -> [_ w1597 w1632]
              tunnel: w1590 -> [_ _ w1630]
              frame 0, Default {
              }
              frame 1 {
                n625 = Unbundle By Name(w1605) -> ("SET VALUE 8"=w1625:dbl, "TOL 8"=w1623:dbl, "RES VALUE 8"=w1621:dbl, "CH  PASS 8"=w1619:bool, "CH8 MAX TOL"=w1604:dbl, "CH8 MIN TOL"=w1602:dbl)
                n626 = case shown="False" w1619 {
                  tunnel: ["FAIL" "PASS"] -> w1612
                  frame False {
                  }
                  frame True {
                  }
                }
                n627 = case shown="True" w1600 {
                  tunnel: ["NORMAL" "RETEST"] -> w1596
                  frame False {
                  }
                  frame True {
                  }
                }
                n628 = Get Date/Time String() -> (date string=w1617:string, time string=w1618:string)  [unwired: 3 in]
                n629 = Concatenate Strings(w1617, w1618) -> (w1616:string)
                n630 = Number To Fractional String(number=w1604, precision (6)=i16 3) -> (F-format string=w1599:string)  [unwired: 2 in]
                n631 = Number To Fractional String(number=w1625, precision (6)=i16 3 ("width (-)")) -> (F-format string=w1615:string)  [unwired: 2 in]
                n632 = Number To Fractional String(number=w1623, precision (6)=i16 3 ("width (-)")) -> (F-format string=w1614:string)  [unwired: 2 in]
                n633 = Number To Fractional String(number=w1621, precision (6)=i16 3 ("width (-)")) -> (F-format string=w1613:string)  [unwired: 2 in]
                n634 = Number To Fractional String(number=w1602, precision (6)=i16 3) -> (F-format string=w1598:string)  [unwired: 2 in]
                n635 = Build Array(w1616, w1615, w1614, w1613, w1612, "8" ("element"), w1599, w1598, w1597, w1596) -> (w1610:string[])
                n636 = call-poly <vilib>:"Write Delimited Spreadsheet.vi"("file path (dialog if empty)"=w1606, "1D data"=w1610, "append to file? (new file:F)"=TRUE, "transpose? (no:F)"=FALSE, "delimiter (\\t)"="," ("delimiter (\\t)")) -> ()  [unwired: 9 in, 2 out]
              }
              frame 2 {
                n637 = case shown="True" w1630 {
                  tunnel: w1634 -> [_ w1638]
                  tunnel: w1633 -> [_ w1637]
                  tunnel: w1632 -> [_ w1636]
                  tunnel: w1631 -> [_ w1635]
                  frame False {
                  }
                  frame True {
                    n638 = Unbundle By Name(w1637) -> ("SET VALUE 8"=w1664:dbl, "TOL 8"=w1662:dbl, "RES VALUE 8"=w1660:dbl, "CH  PASS 8"=w1658:bool, "CH8 MAX TOL"=w1645:dbl, "CH8 MIN TOL"=w1643:dbl)
                    n639 = case shown="False" w1658 {
                      tunnel: ["FAIL" "PASS"] -> w1651
                      frame False {
                      }
                      frame True {
                      }
                    }
                    n640 = case shown="True" w1635 {
                      tunnel: ["NORMAL" "RETEST"] -> w1639
                      frame False {
                      }
                      frame True {
                      }
                    }
                    n641 = Get Date/Time String() -> (date string=w1656:string, time string=w1657:string)  [unwired: 3 in]
                    n642 = Concatenate Strings(w1656, w1657) -> (w1655:string)
                    n643 = Number To Fractional String(number=w1645, precision (6)=i16 3) -> (F-format string=w1641:string)  [unwired: 2 in]
                    n644 = Number To Fractional String(number=w1664, precision (6)=i16 3 ("width (-)")) -> (F-format string=w1654:string)  [unwired: 2 in]
                    n645 = Number To Fractional String(number=w1662, precision (6)=i16 3 ("width (-)")) -> (F-format string=w1653:string)  [unwired: 2 in]
                    n646 = Number To Fractional String(number=w1660, precision (6)=i16 3 ("width (-)")) -> (F-format string=w1652:string)  [unwired: 2 in]
                    n647 = Number To Fractional String(number=w1643, precision (6)=i16 3) -> (F-format string=w1640:string)  [unwired: 2 in]
                    n648 = Build Array(w1655, w1654, w1653, w1652, w1651, "8" ("element"), w1641, w1640, w1636, w1639) -> (w1649:string[])
                    n649 = call-poly <vilib>:"Write Delimited Spreadsheet.vi"("file path (dialog if empty)"=w1638, "1D data"=w1649, "append to file? (new file:F)"=TRUE, "transpose? (no:F)"=FALSE, "delimiter (\\t)"="," ("delimiter (\\t)")) -> ()  [unwired: 9 in, 2 out]
                  }
                }
              }
            }
          }
          frame #8 {
            # "Channel 9 data log"
            n650 = Unbundle By Name(w1673) -> ("PP 9"=w1674:i32)
            n651 = case shown="2" w1674 {
              tunnel: w1673 -> [_ w1684 w1709]
              tunnel: w1672 -> [_ w1685 w1713]
              tunnel: w1671 -> [_ w1677 w1710]
              tunnel: w1670 -> [_ w1675 w1711]
              tunnel: w1669 -> [_ _ w1712]
              frame 0, Default {
              }
              frame 1 {
                n652 = Unbundle By Name(w1684) -> ("SET VALUE 9"=w1704:dbl, "TOL 9"=w1702:dbl, "RES VALUE 9"=w1700:dbl, "CH  PASS 9"=w1698:bool, "CH9 MAX TOL"=w1683:dbl, "CH9 MIN TOL"=w1682:dbl)
                n653 = case shown="False" w1698 {
                  tunnel: ["FAIL" "PASS"] -> w1691
                  frame False {
                  }
                  frame True {
                  }
                }
                n654 = case shown="False" w1677 {
                  tunnel: ["NORMAL" "RETEST"] -> w1676
                  frame False {
                  }
                  frame True {
                  }
                }
                n655 = Get Date/Time String() -> (date string=w1696:string, time string=w1697:string)  [unwired: 3 in]
                n656 = Concatenate Strings(w1696, w1697) -> (w1695:string)
                n657 = Number To Fractional String(number=w1683, precision (6)=i16 3) -> (F-format string=w1679:string)  [unwired: 2 in]
                n658 = Number To Fractional String(number=w1704, precision (6)=i16 3 ("width (-)")) -> (F-format string=w1694:string)  [unwired: 2 in]
                n659 = Number To Fractional String(number=w1702, precision (6)=i16 3 ("width (-)")) -> (F-format string=w1693:string)  [unwired: 2 in]
                n660 = Number To Fractional String(number=w1700, precision (6)=i16 3 ("width (-)")) -> (F-format string=w1692:string)  [unwired: 2 in]
                n661 = Number To Fractional String(number=w1682, precision (6)=i16 3) -> (F-format string=w1678:string)  [unwired: 2 in]
                n662 = Build Array(w1695, w1694, w1693, w1692, w1691, "9" ("element"), w1679, w1678, w1675, w1676) -> (w1689:string[])
                n663 = call-poly <vilib>:"Write Delimited Spreadsheet.vi"("file path (dialog if empty)"=w1685, "1D data"=w1689, "append to file? (new file:F)"=TRUE, "transpose? (no:F)"=FALSE, "delimiter (\\t)"="," ("delimiter (\\t)")) -> ()  [unwired: 9 in, 2 out]
              }
              frame 2 {
                n664 = case shown="True" w1712 {
                  tunnel: w1713 -> [_ w1717]
                  tunnel: w1711 -> [_ w1716]
                  tunnel: w1710 -> [_ w1715]
                  tunnel: w1709 -> [_ w1714]
                  frame False {
                  }
                  frame True {
                    n665 = Unbundle By Name(w1714) -> ("SET VALUE 9"=w1743:dbl, "TOL 9"=w1741:dbl, "RES VALUE 9"=w1739:dbl, "CH  PASS 9"=w1737:bool, "CH9 MAX TOL"=w1724:dbl, "CH9 MIN TOL"=w1723:dbl)
                    n666 = case shown="False" w1737 {
                      tunnel: ["FAIL" "PASS"] -> w1730
                      frame False {
                      }
                      frame True {
                      }
                    }
                    n667 = case shown="False" w1715 {
                      tunnel: ["NORMAL" "RETEST"] -> w1718
                      frame False {
                      }
                      frame True {
                      }
                    }
                    n668 = Get Date/Time String() -> (date string=w1735:string, time string=w1736:string)  [unwired: 3 in]
                    n669 = Concatenate Strings(w1735, w1736) -> (w1734:string)
                    n670 = Number To Fractional String(number=w1724, precision (6)=i16 3) -> (F-format string=w1720:string)  [unwired: 2 in]
                    n671 = Number To Fractional String(number=w1743, precision (6)=i16 3 ("width (-)")) -> (F-format string=w1733:string)  [unwired: 2 in]
                    n672 = Number To Fractional String(number=w1741, precision (6)=i16 3 ("width (-)")) -> (F-format string=w1732:string)  [unwired: 2 in]
                    n673 = Number To Fractional String(number=w1739, precision (6)=i16 3 ("width (-)")) -> (F-format string=w1731:string)  [unwired: 2 in]
                    n674 = Number To Fractional String(number=w1723, precision (6)=i16 3) -> (F-format string=w1719:string)  [unwired: 2 in]
                    n675 = Build Array(w1734, w1733, w1732, w1731, w1730, "9" ("element"), w1720, w1719, w1716, w1718) -> (w1728:string[])
                    n676 = call-poly <vilib>:"Write Delimited Spreadsheet.vi"("file path (dialog if empty)"=w1717, "1D data"=w1728, "append to file? (new file:F)"=TRUE, "transpose? (no:F)"=FALSE, "delimiter (\\t)"="," ("delimiter (\\t)")) -> ()  [unwired: 9 in, 2 out]
                  }
                }
              }
            }
          }
          frame #9 {
            # "Channel 10 data log"
            n677 = Unbundle By Name(w1752) -> ("PP 10"=w1753:i32)
            n678 = case shown="2" w1753 {
              tunnel: w1752 -> [_ w1763 w1791]
              tunnel: w1751 -> [_ w1764 w1792]
              tunnel: w1750 -> [_ w1758 w1789]
              tunnel: w1749 -> [_ w1755 w1790]
              tunnel: w1748 -> [_ _ w1788]
              frame 0, Default {
              }
              frame 1 {
                n679 = Unbundle By Name(w1763) -> ("SET VALUE 10"=w1783:dbl, "TOL 10"=w1781:dbl, "RES VALUE 10"=w1779:dbl, "CH  PASS 10"=w1777:bool, "CH10 MAX TOL"=w1762:dbl, "CH10 MIN TOL"=w1761:dbl)
                n680 = case shown="False" w1777 {
                  tunnel: ["FAIL" "PASS"] -> w1770
                  frame False {
                  }
                  frame True {
                  }
                }
                n681 = case shown="True" w1758 {
                  tunnel: ["NORMAL" "RETEST"] -> w1754
                  frame False {
                  }
                  frame True {
                  }
                }
                n682 = Get Date/Time String() -> (date string=w1775:string, time string=w1776:string)  [unwired: 3 in]
                n683 = Concatenate Strings(w1775, w1776) -> (w1774:string)
                n684 = Number To Fractional String(number=w1762, precision (6)=i16 3) -> (F-format string=w1760:string)  [unwired: 2 in]
                n685 = Number To Fractional String(number=w1783, precision (6)=i16 3 ("width (-)")) -> (F-format string=w1773:string)  [unwired: 2 in]
                n686 = Number To Fractional String(number=w1781, precision (6)=i16 3 ("width (-)")) -> (F-format string=w1772:string)  [unwired: 2 in]
                n687 = Number To Fractional String(number=w1779, precision (6)=i16 3 ("width (-)")) -> (F-format string=w1771:string)  [unwired: 2 in]
                n688 = Number To Fractional String(number=w1761, precision (6)=i16 3) -> (F-format string=w1759:string)  [unwired: 2 in]
                n689 = Build Array(w1774, w1773, w1772, w1771, w1770, "10" ("element"), w1760, w1759, w1755, w1754) -> (w1768:string[])
                n690 = call-poly <vilib>:"Write Delimited Spreadsheet.vi"("file path (dialog if empty)"=w1764, "1D data"=w1768, "append to file? (new file:F)"=TRUE, "transpose? (no:F)"=FALSE, "delimiter (\\t)"="," ("delimiter (\\t)")) -> ()  [unwired: 9 in, 2 out]
              }
              frame 2 {
                n691 = case shown="True" w1788 {
                  tunnel: w1792 -> [_ w1796]
                  tunnel: w1791 -> [_ w1795]
                  tunnel: w1790 -> [_ w1794]
                  tunnel: w1789 -> [_ w1793]
                  frame False {
                  }
                  frame True {
                    n692 = Unbundle By Name(w1795) -> ("SET VALUE 10"=w1822:dbl, "TOL 10"=w1820:dbl, "RES VALUE 10"=w1818:dbl, "CH  PASS 10"=w1816:bool, "CH10 MAX TOL"=w1803:dbl, "CH10 MIN TOL"=w1802:dbl)
                    n693 = case shown="False" w1816 {
                      tunnel: ["FAIL" "PASS"] -> w1809
                      frame False {
                      }
                      frame True {
                      }
                    }
                    n694 = case shown="True" w1793 {
                      tunnel: ["NORMAL" "RETEST"] -> w1797
                      frame False {
                      }
                      frame True {
                      }
                    }
                    n695 = Get Date/Time String() -> (date string=w1814:string, time string=w1815:string)  [unwired: 3 in]
                    n696 = Concatenate Strings(w1814, w1815) -> (w1813:string)
                    n697 = Number To Fractional String(number=w1803, precision (6)=i16 3) -> (F-format string=w1801:string)  [unwired: 2 in]
                    n698 = Number To Fractional String(number=w1822, precision (6)=i16 3 ("width (-)")) -> (F-format string=w1812:string)  [unwired: 2 in]
                    n699 = Number To Fractional String(number=w1820, precision (6)=i16 3 ("width (-)")) -> (F-format string=w1811:string)  [unwired: 2 in]
                    n700 = Number To Fractional String(number=w1818, precision (6)=i16 3 ("width (-)")) -> (F-format string=w1810:string)  [unwired: 2 in]
                    n701 = Number To Fractional String(number=w1802, precision (6)=i16 3) -> (F-format string=w1800:string)  [unwired: 2 in]
                    n702 = Build Array(w1813, w1812, w1811, w1810, w1809, "10" ("element"), w1801, w1800, w1794, w1797) -> (w1807:string[])
                    n703 = call-poly <vilib>:"Write Delimited Spreadsheet.vi"("file path (dialog if empty)"=w1796, "1D data"=w1807, "append to file? (new file:F)"=TRUE, "transpose? (no:F)"=FALSE, "delimiter (\\t)"="," ("delimiter (\\t)")) -> ()  [unwired: 9 in, 2 out]
                  }
                }
              }
            }
          }
        }
      }
      frame "PART PRESENCE CHECKING" {
      }
    }
  }
